vi "Initialize_etc.vi"(7 "큐 입력":refnum<queue>, 8 "error in":errorcluster caption="에러 입력(에러 없음)", 11 "입력 클러스터":T1) -> (0 "error out":errorcluster caption="에러 출력", 3 "data 1":string[][](array[string]), 4 "Load?":bool)   [LabVIEW 2020]
uses:
  Controls/Clst_Initialize Input.ctl
  Controls/Cmd_Var Data IO.ctl
  Variables/Global_Cal Info.vi
  Public/Polymorph/Table Initialize_2D.vi
  Public/Polymorph/Array Dedup_1D Str.vi
  Public/Polymorph/String content_Str.vi
  Public/Polymorph/String content_Combo.vi
  Public/Polymorph/Table Initialize_Str.vi
  Public/Polymorph/Cell Space_Table.vi
  Public/Polymorph/Rmv Empt Arr_2D Str.vi
  <vilib>/express/express arith-compare/Formula/XNode/ExpressFormulaBlockNode.xnode
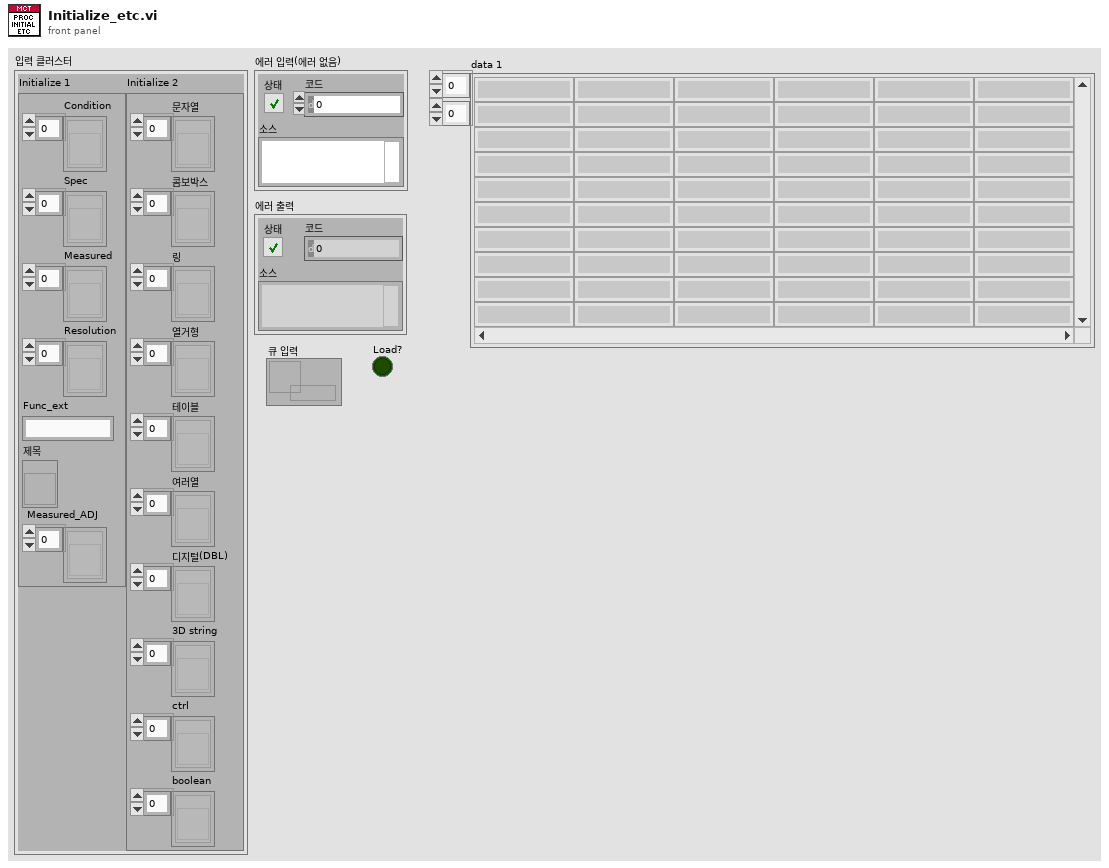
[diagram p1: front panel]
types:
  T1 = typedef "Clst_Initialize Input.ctl" = cluster{"Initialize 1":cluster{"Condition":refnum<vi>[], "Spec":refnum<vi>[], "Measured":refnum<vi>[], "Resolution":refnum<vi>[], "Func_ext":string, "제목":refnum<vi>, "Measured_ADJ":refnum<vi>[]}, "Initialize 2":cluster{"문자열":refnum<vi>[], "콤보박스":refnum<vi>[], "링":refnum<vi>[], "열거형":refnum<vi>[], "테이블":refnum<vi>[], "여러열":refnum<vi>[], "디지털(DBL)":refnum<vi>[], "3D string":refnum<vi>[], "ctrl":refnum<vi>[], "boolean":refnum<vi>[]}}
  T2 = cluster{"세부분류코드":string, "형식":string, "옵션":string, "측정기명":string, "EXCEL파일명":string, "TEMP":string}
  T3 = typedef "Cmd_Var Data IO.ctl" = enum16{"Condition", "Condition Default", "Condition_Temp", "Resolution", "Resolution Default", "Resolution Old", "Spec", "Spec Default", "Spec Old", "Spec Temp", "Result", "Result2", "Result3", "Result_Temp", "Result_ADJ", "Result_ADJ2", "STD1", "STD2", "STD3", "STD4", "STD5", "STD Temp", "CMC", "CMC Default"}
  T4 = enum8{"Enabled", "Disabled", "Disabled and Grayed Out"}
  T5 = typedef "Clst_Get Calproc.ctl" = cluster{"제목":string, "Condition":string[][], "Resolution":string[][], "Spec":string[][], "Data":string[][], "CMC":string[][], "NumRows":u32, "Temp_1":string[][]}
  T6 = typedef "Clst_Atm Info Global.ctl" = cluster{"교정장소":enum16{"0 : 고정표준실", "1 : 현장교정"}, "최저온도(℃)":string, "최고온도(℃)":string, "최저습도(％ R.H.)":string, "최고습도(％ R.H.)":string, "최저기압(hPa)":string, "최고기압(hPa)":string, "교정실명":string}
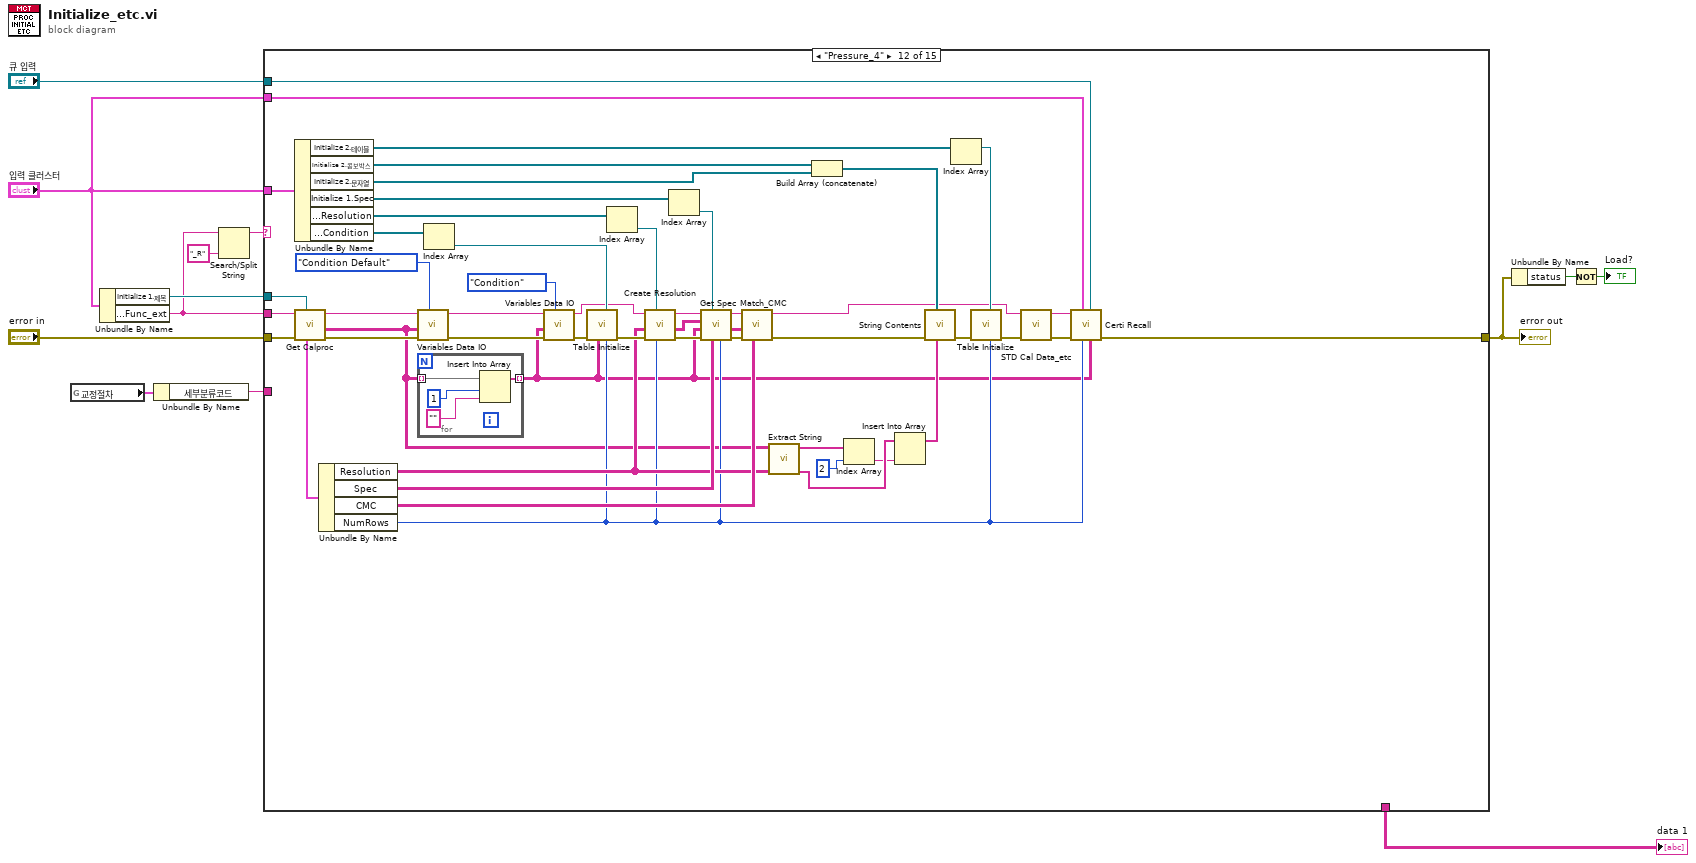
[diagram p0: block diagram]
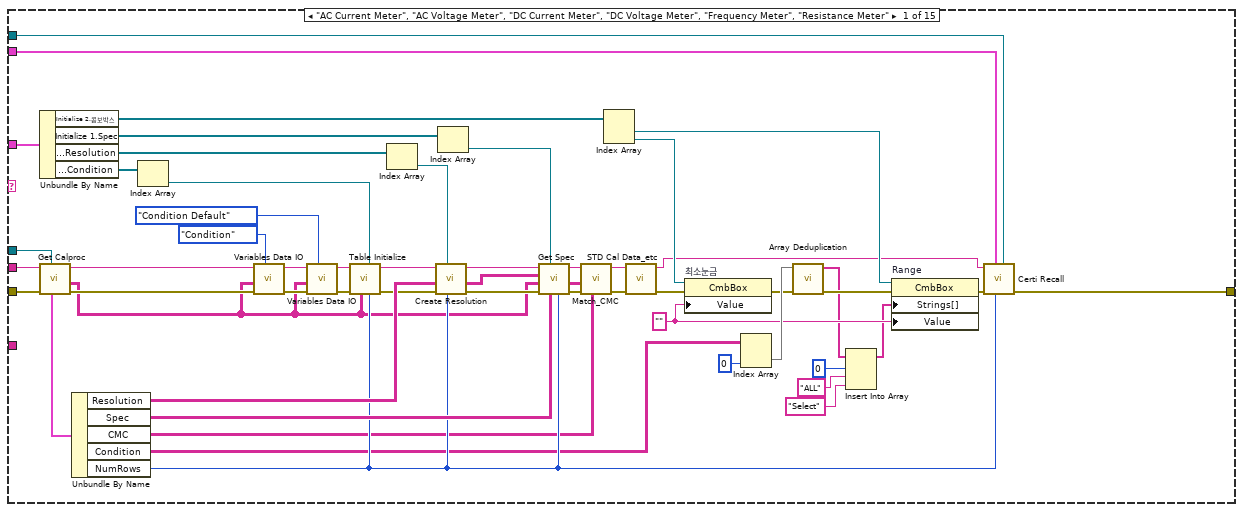
[diagram p2: hidden frame]
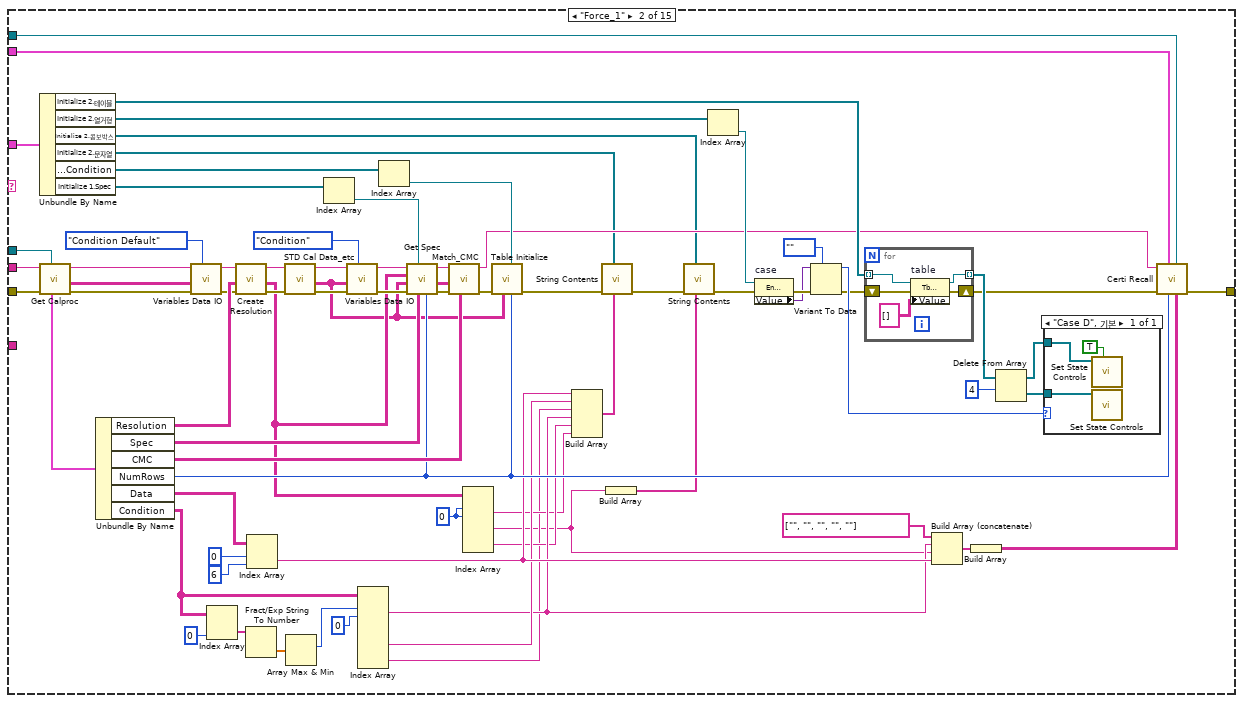
[diagram p3: hidden frame]
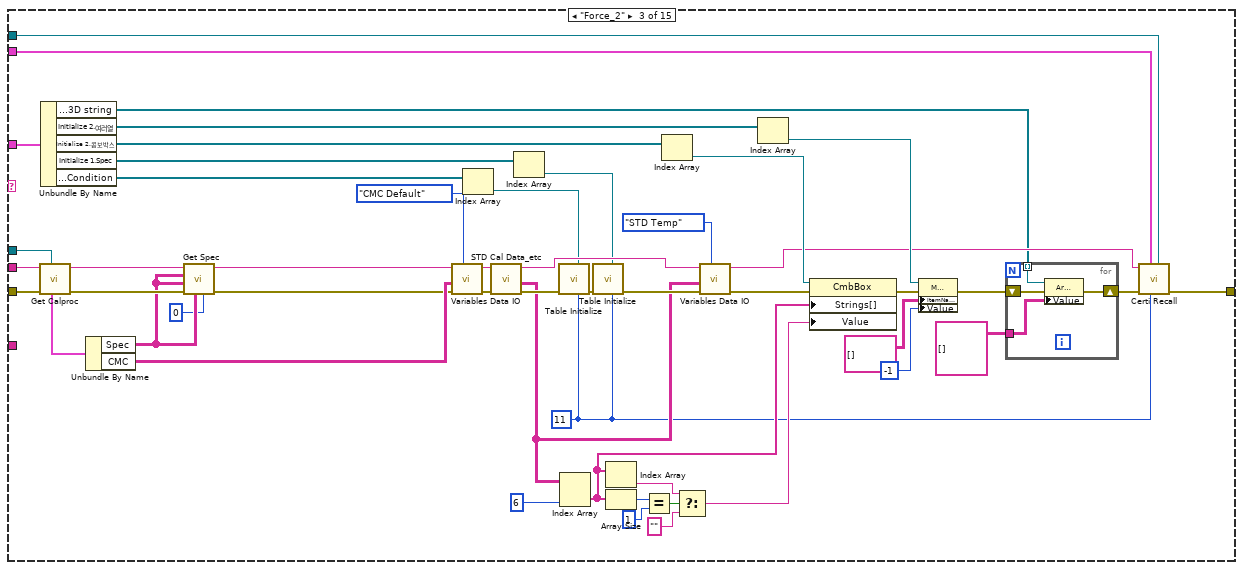
[diagram p4: hidden frame]
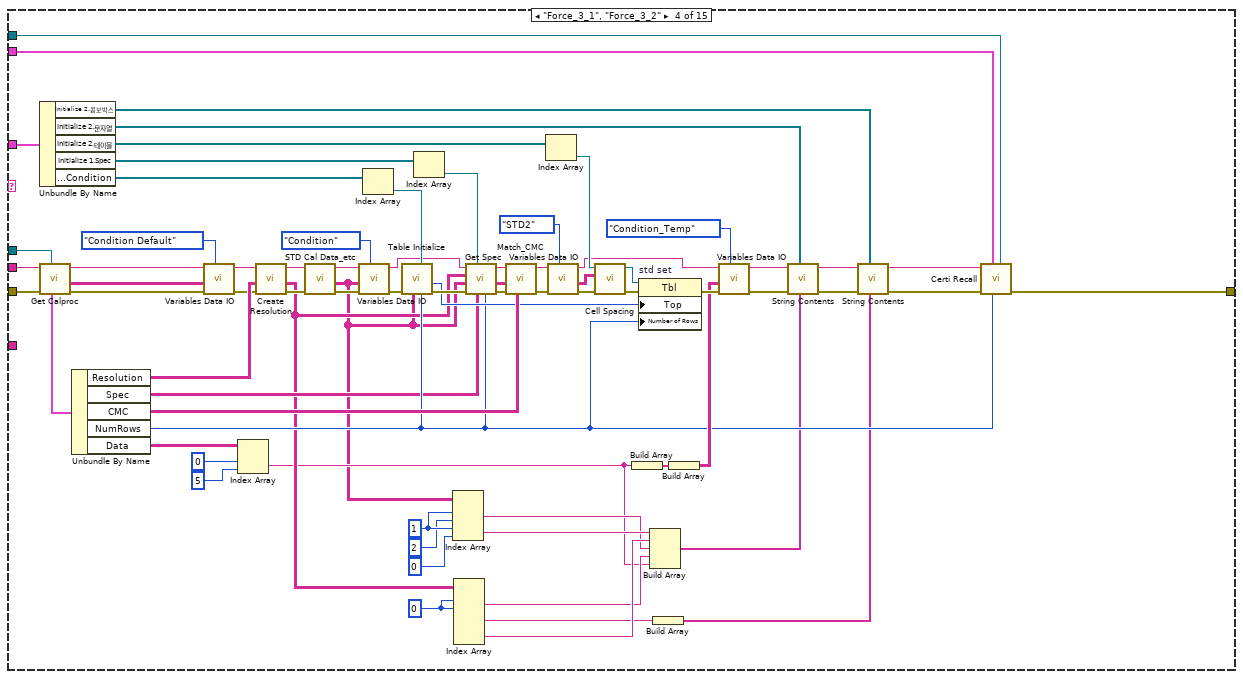
[diagram p5: hidden frame]
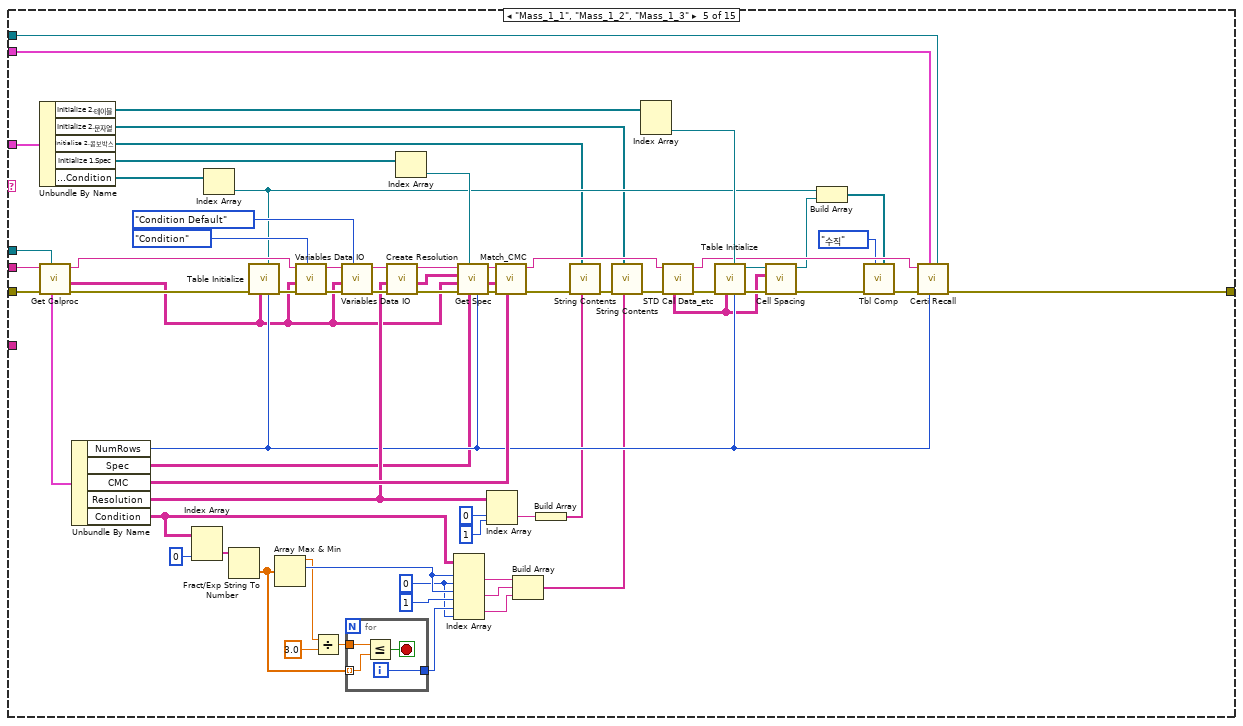
[diagram p6: hidden frame]
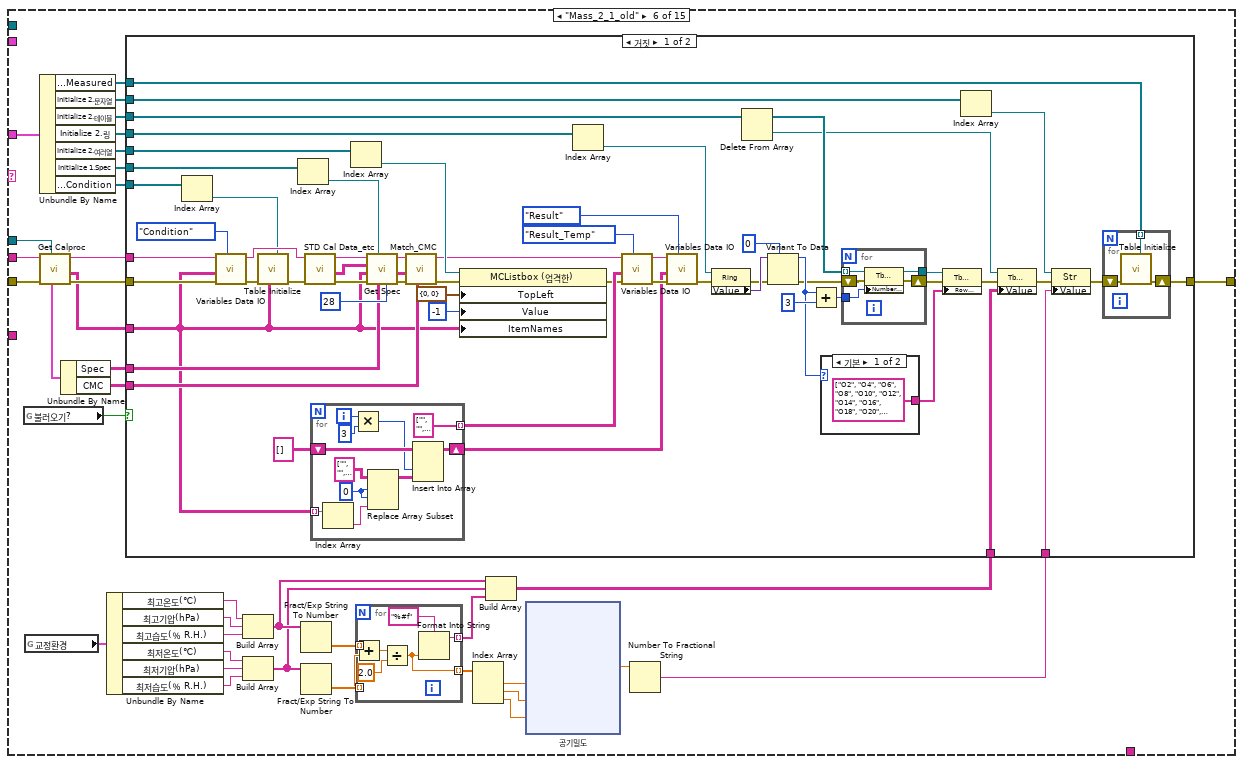
[diagram p7: hidden frame]
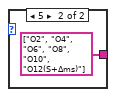
[diagram p8: hidden frame]
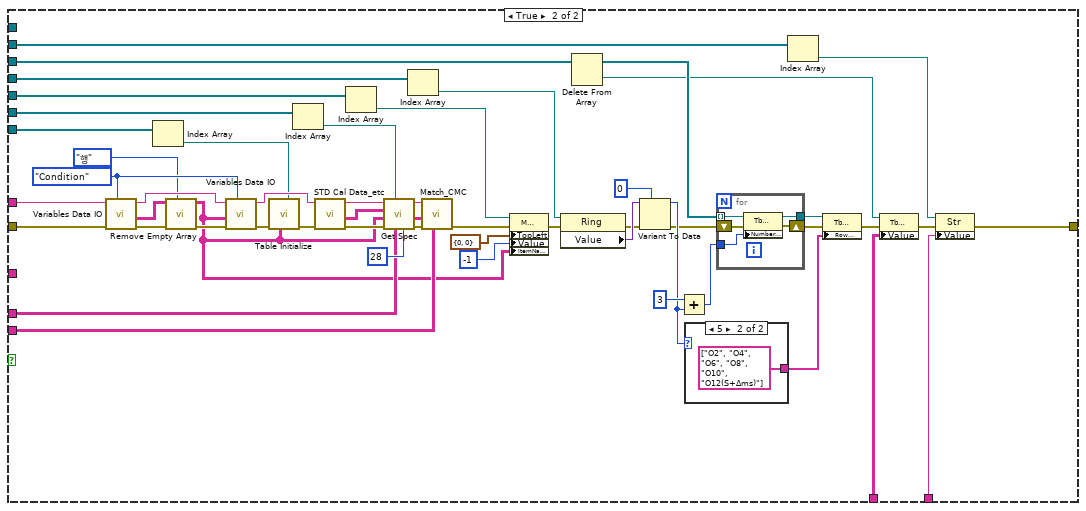
[diagram p9: hidden frame]
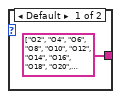
[diagram p10: hidden frame]
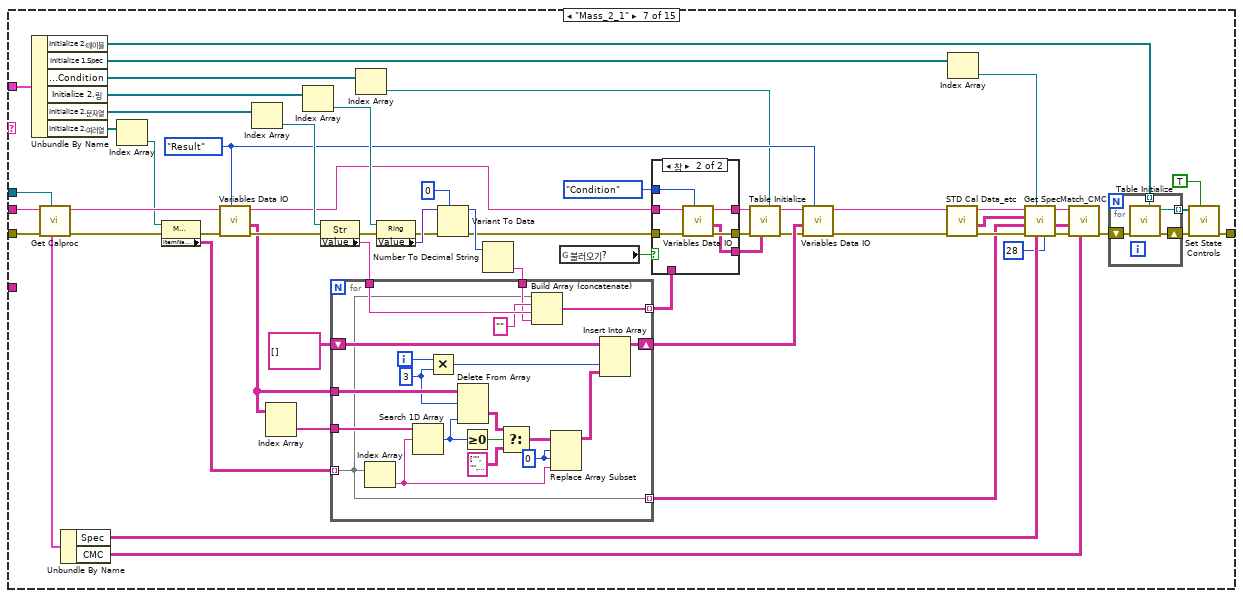
[diagram p11: hidden frame]
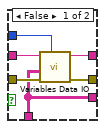
[diagram p12: hidden frame]
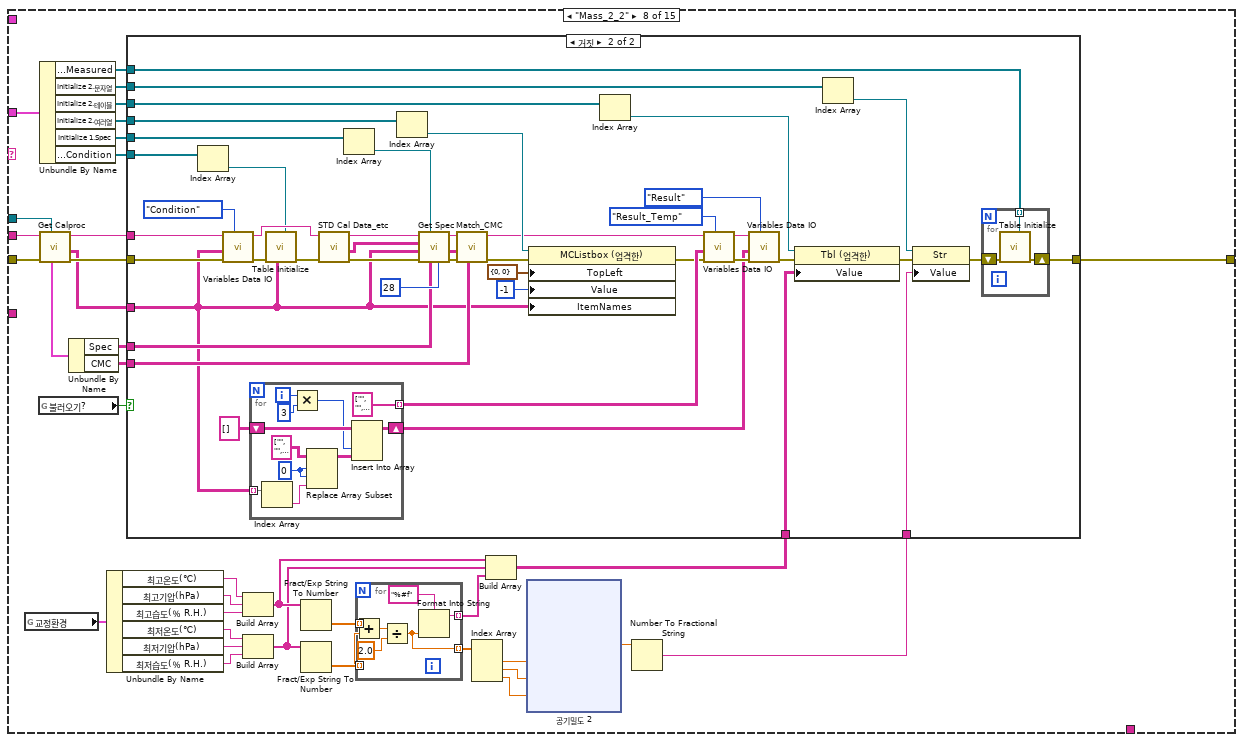
[diagram p13: hidden frame]
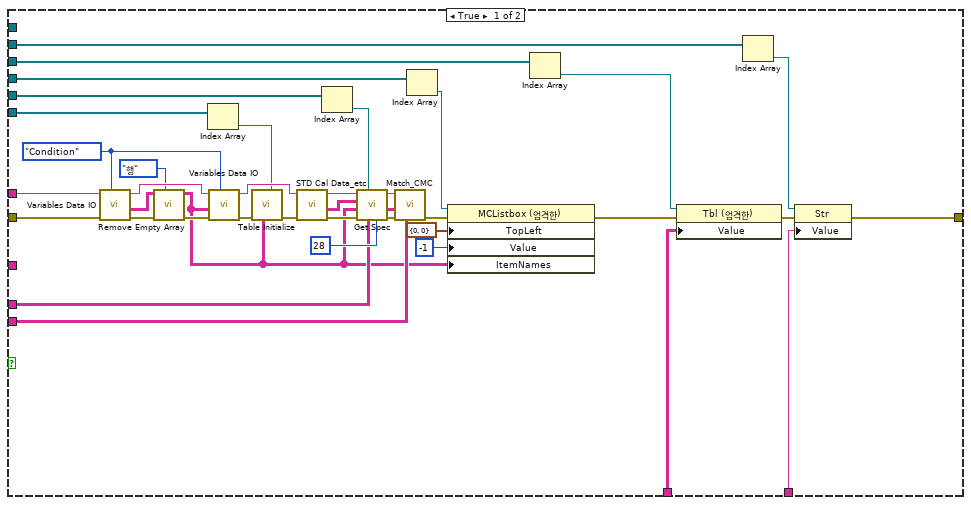
[diagram p14: hidden frame]
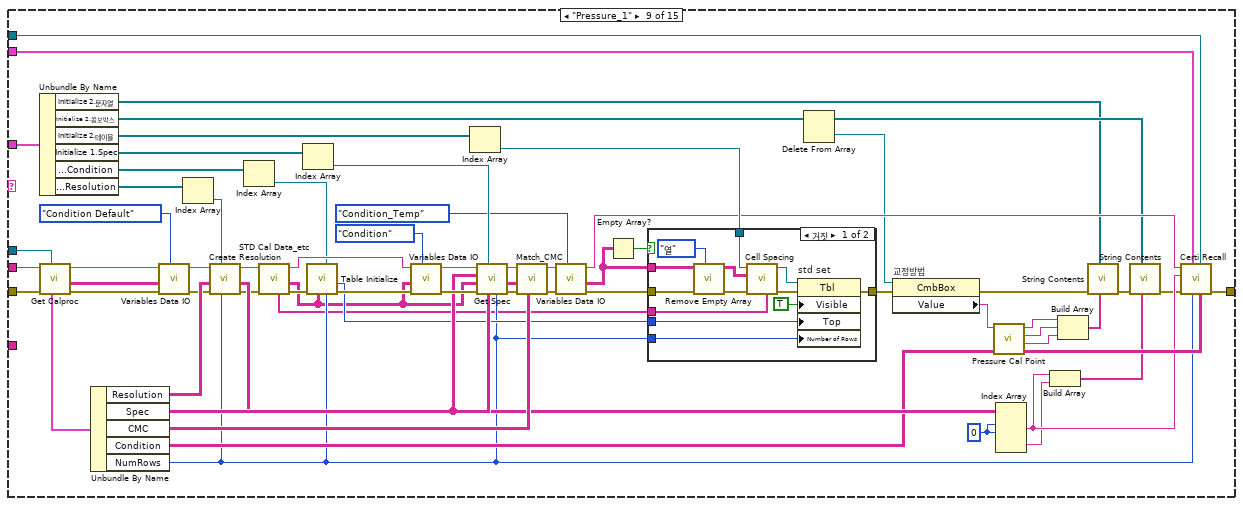
[diagram p15: hidden frame]
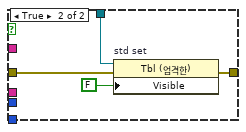
[diagram p16: hidden frame]
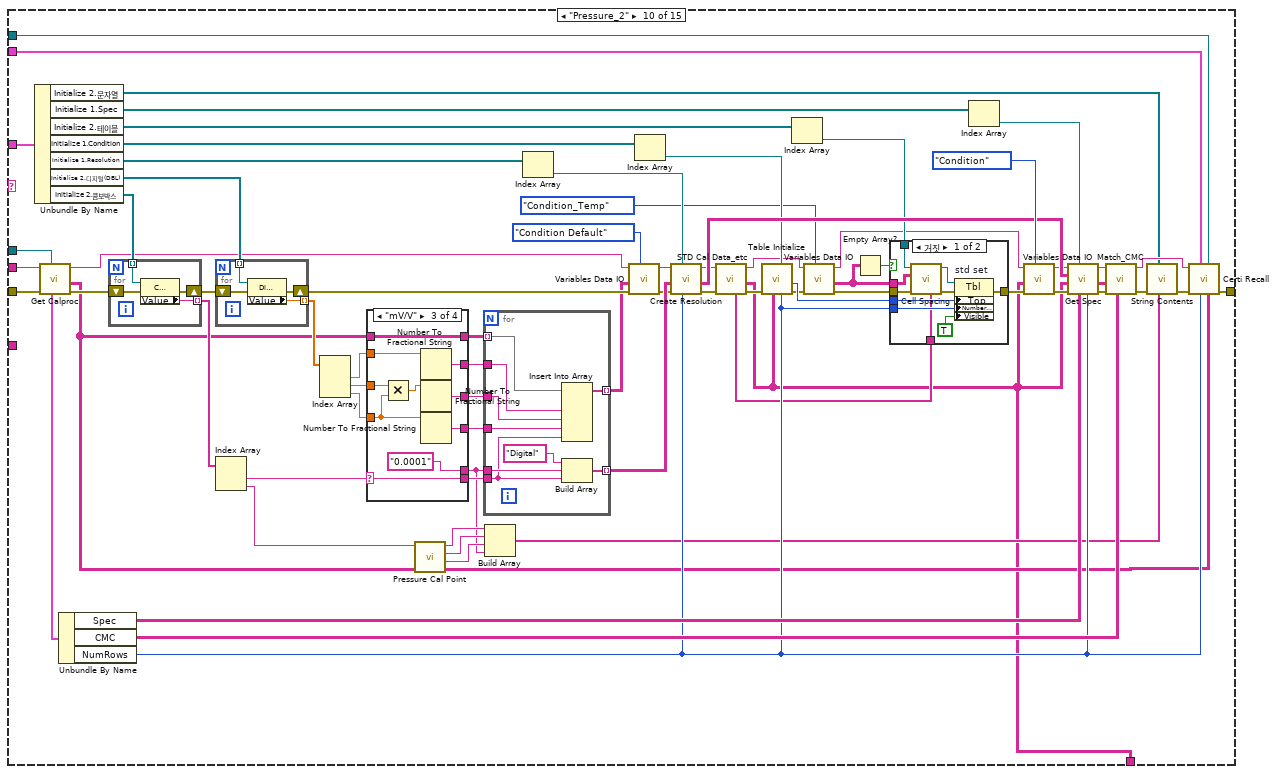
[diagram p17: hidden frame]
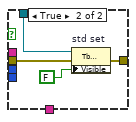
[diagram p18: hidden frame]
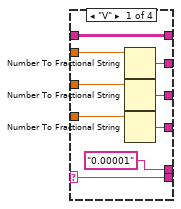
[diagram p19: hidden frame]
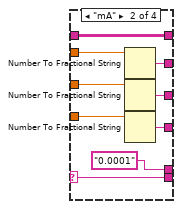
[diagram p20: hidden frame]
diagram:
  n1 = global read "Global_Cal Info.vi" "교정절차"() -> (w11:T2)
  n2 = Unbundle By Name("입력 클러스터") -> ("Initialize 1.제목"=w9:refnum<vi>, "Initialize 1.Func_ext"=w4:string)
  n3 = Unbundle By Name(w11) -> ("세부분류코드"=w10:string)
  n4 = Search/Split String(string=w4, search string/char (-)="_R" ("검색 문자열/문자 (-)")) -> (substring before match=w3:string)  [unwired: 1 in, 2 out]
  n5 = case shown="\"Pressure_4\"" w3 {
    tunnel: "error in" -> [w66 w141 w199 w274 w342 w384 w601 w674 w858 w949 w1090 w1140 w1205 w1271 w1287]
    tunnel: [w25 w74 w163 w225 w307 w360 w590 w651 w837 w917 w1063 w1128 w1174 w1257 w1287] -> w8
    tunnel: "입력 클러스터" -> [w24 w115 w170 w244 w343 w385 w602 w675 w859 w950 w1091 w1141 w1206 w1272 _]
    tunnel: [_ _ _ _ _ _ _ _ _ w877 _ _ _ w1207 string[][] [] ("CMC Out")] -> w13
    tunnel: "큐 입력" -> [w34 w104 w165 w227 w306 _ _ _ w836 w930 w1066 w1130 w1173 w1258 _]
    tunnel: w4 -> [w37 w133 w198 w263 w311 w354 w594 w645 w840 w937 w1075 w1133 w1194 w1260 _]
    tunnel: w10 -> [_ _ _ _ _ _ _ _ _ _ _ _ _ _ _]
    tunnel: "입력 클러스터" -> [w23 w103 w164 w226 w305 _ _ _ w835 w929 w1064 w1129 w1172 w1256 _]
    tunnel: w9 -> [w18 w89 w161 w218 w298 w352 w592 w643 w824 w921 w1054 w1125 w1163 w1253 _]
    frame "AC Current Meter", "AC Voltage Meter", "DC Current Meter", "DC Voltage Meter", "Frequency Meter", "Resistance Meter" {
      w51 = "" ("값")
      n6 = Unbundle By Name(w24) -> ("Initialize 2.콤보박스"=w63:refnum<vi>[], "Initialize 1.Spec"=w28:refnum<vi>[], "Initialize 1.Resolution"=w29:refnum<vi>[], "Initialize 1.Condition"=w65:refnum<vi>[])
      n7 = call "Get Calproc.vi"("제목"=w18, "에러 입력"=w66, "Func_ext"=w37) -> ("에러 출력"=w64:errorcluster, "Condition"=w14:string[][], "Func_ext Out"=w39:string, "클러스터"=w32:T5)  [unwired: 5 in]
      n8 = Unbundle By Name(w32) -> ("Resolution"=w40:string[][], "Spec"=w22:string[][], "CMC"=w16:string[][], "Condition"=w15:string[][], "NumRows"=w17:u32)
      n9 = Index Array(array=w65) -> (element=w35:refnum<vi>)  [unwired: 1 in]
      n10 = call "Variables Data IO.vi"("Select"=Cmd_Var_Data_IO."Condition", "error in"=w64, "Data In"=w14, "Func_ext"=w39) -> ("error out"=w61:errorcluster, "Func_ext Out"=w43:string)  [unwired: 5 in, 1 out]
      n11 = call "Variables Data IO.vi"("Select"=Cmd_Var_Data_IO."Condition Default", "error in"=w61, "Data In"=w14, "Func_ext"=w43) -> ("error out"=w31:errorcluster, "Func_ext Out"=w42:string)  [unwired: 5 in, 1 out]
      n12 = call-poly "Table Initialize.vi"("행의 개수"=w17, "Table Ref"=w35, "Value"=w14, "에러 입력"=w31) -> ("에러 출력"=w30:errorcluster)  [unwired: 5 in, 2 out]
      n13 = Index Array(array=w29) -> (element=w19:refnum<vi>)  [unwired: 1 in]
      n14 = call "Create Resolution.vi"("행의 개수"=w17, "Table Ref"=w19, "에러 입력(에러 없음)"=w30, "Resolution"=w40, "Func_ext"=w42) -> ("에러 출력"=w44:errorcluster, "Resolution Out"=w21:string[][], "Func_ext 출력"=w20:string)  [unwired: 4 in]
      n15 = Index Array(array=w28) -> (element=w50:refnum<vi>)  [unwired: 1 in]
      n16 = call "Get Spec.vi"("NumRows"=w17, "Spec in"=w22, "Spec Ref."=w50, "error in"=w44, "Condition in"=w14, "Resolution in"=w21, "Func_ext"=w20) -> ("error out"=w59:errorcluster, "Data Out"=w36:string[][], "Func_ext Out"=w41:string)  [unwired: 2 out]
      n17 = call "Match_CMC.vi"("CMC IN"=w16, "error in"=w59, "Condition IN"=w36, "Func_ext"=w41) -> ("error out"=w58:errorcluster, "Func_ext out"=w38:string)  [unwired: 4 in, 2 out]
      n18 = Index Array(array=w63) -> (element #1=w55:refnum<vi>, element #2=w57:refnum<vi>)  [unwired: 2 in]
      n19 = call "STD Cal Data_etc.vi"("error in"=w58, "Func_ext"=w38) -> ("error out"=w27:errorcluster, "Func_ext Out"=w33:string)  [unwired: 5 in, 3 out]
      n20 = property on="최소눈금" class="CmbBox"(reference=w57, error in=w27, "Value"=w51) -> (error out=w53:errorcluster)  [unwired: 1 out]
      n21 = Index Array(array=w15, index (col)=0 ("비활성화된 인덱스 (열)")) -> (element=w54:string[])  [unwired: 1 in]
      n22 = call-poly "Array Deduplication.vi"("error in (no error)"=w53, "배열 in"=w54) -> ("error out"=w52:errorcluster, "배열 out"=w46:string[])  [unwired: 8 in]
      n23 = Insert Into Array(array=w46, index=0 ("인덱스"), new element #1="ALL" ("새 원소/부분배열"), new element #2="Select" ("새 원소/부분배열")) -> (w45:string[])
      n24 = property on="Range" class="CmbBox"(reference=w55, error in=w52, "Strings[]"=w45, "Value"=w51) -> (error out=w26:errorcluster)  [unwired: 1 out]
      n25 = call "Certi Recall.vi"("큐 입력"=w34, "NumRows"=w17, "입력 클러스터"=w23, "에러 입력"=w26, "Func_ext in"=w33) -> ("에러 출력"=w25:errorcluster)  [unwired: 5 in, 1 out]
    }
    frame "Force_1" {
      w111 = 0 ("인덱스 (행)")
      n26 = Unbundle By Name(w115) -> ("Initialize 2.테이블"=w112:refnum<vi>[], "Initialize 2.열거형"=w100:refnum<vi>[], "Initialize 2.콤보박스"=w68:refnum<vi>[], "Initialize 2.문자열"=w76:refnum<vi>[], "Initialize 1.Condition"=w131:refnum<vi>[], "Initialize 1.Spec"=w96:refnum<vi>[])
      n27 = call "Get Calproc.vi"("제목"=w89, "에러 입력"=w141, "Func_ext"=w133) -> ("에러 출력"=w140:errorcluster, "Condition"=w88:string[][], "Func_ext Out"=w136:string, "클러스터"=w107:T5)  [unwired: 5 in]
      n28 = Unbundle By Name(w107) -> ("Resolution"=w130:string[][], "Spec"=w92:string[][], "CMC"=w135:string[][], "NumRows"=w98:u32, "Data"=w110:string[][], "Condition"=w87:string[][])
      n29 = call "Variables Data IO.vi"("Select"=Cmd_Var_Data_IO."Condition Default", "error in"=w140, "Data In"=w88, "Func_ext"=w136) -> ("error out"=w129:errorcluster, "Func_ext Out"=w126:string)  [unwired: 5 in, 1 out]
      n30 = Index Array(array=w87, index (col)=0 ("비활성화된 인덱스 (열)")) -> (element=w122:string[])  [unwired: 1 in]
      n31 = call "Create Resolution.vi"("에러 입력(에러 없음)"=w129, "Resolution"=w130, "Func_ext"=w126) -> ("에러 출력"=w128:errorcluster, "Resolution Out"=w91:string[][], "Func_ext 출력"=w125:string)  [unwired: 6 in]
      n32 = Fract/Exp String To Number(string=w122) -> (number=w121:dbl[])  [unwired: 3 in, 1 out]
      n33 = Index Array(array=w110, index (row)=0 ("인덱스 (행)"), index (col)=6 ("비활성화된 인덱스 (열)")) -> (element=w82:string)
      n34 = call "STD Cal Data_etc.vi"("error in"=w128, "Func_ext"=w125) -> ("error out"=w127:errorcluster, "Data Out"=w72:string[][], "Func_ext Out"=w124:string)  [unwired: 5 in, 2 out]
      n35 = Array Max & Min(array=w121) -> (max index (indices)=w120:i32)  [unwired: 3 out]
      n36 = Index Array(array=w96) -> (element=w138:refnum<vi>)  [unwired: 1 in]
      n37 = call "Variables Data IO.vi"("Select"=Cmd_Var_Data_IO."Condition", "error in"=w127, "Data In"=w72, "Func_ext"=w124) -> ("error out"=w97:errorcluster, "Func_ext Out"=w90:string)  [unwired: 5 in, 1 out]
      n38 = Index Array(array=w87, index (row) #1=w120, index (col) #1=0 ("비활성화된 인덱스 (열)")) -> (element #1=w80:string, element #3=w81:string, element #4=w75:string)  [unwired: 6 in, 1 out]
      n39 = Index Array(array=w131) -> (element=w123:refnum<vi>)  [unwired: 1 in]
      n40 = call "Get Spec.vi"("NumRows"=w98, "Spec in"=w92, "Spec Ref."=w138, "error in"=w97, "Condition in"=w72, "Resolution in"=w91, "Func_ext"=w90) -> ("error out"=w95:errorcluster, "Data Out"=w132:string[][], "Func_ext Out"=w137:string)  [unwired: 2 out]
      n41 = call "Match_CMC.vi"("CMC IN"=w135, "error in"=w95, "Condition IN"=w132, "Func_ext"=w137) -> ("error out"=w94:errorcluster, "Func_ext out"=w102:string)  [unwired: 4 in, 2 out]
      n42 = Index Array(array=w91, index (row) #1=w111, index (col) #1=w111) -> (element #1=w78:string, element #2=w71:string, element #3=w79:string)  [unwired: 4 in]
      n43 = call-poly "Table Initialize.vi"("행의 개수"=w98, "Table Ref"=w123, "Value"=w72, "에러 입력"=w94) -> ("에러 출력"=w93:errorcluster)  [unwired: 5 in, 2 out]
      n44 = Build Array(w82, w81, w75, w80, w79, w78) -> (w77:string[])
      n45 = call-poly "String Contents.vi"("문자 배열"=w77, "참조 배열"=w76, "에러 입력"=w93) -> ("에러 출력"=w70:errorcluster)  [unwired: 7 in, 1 out]
      n46 = Build Array(w71) -> (w67:string[])
      n47 = call-poly "String Contents.vi"("문자 배열"=w67, "참조 배열"=w68, "에러 입력"=w70) -> ("에러 출력"=w69:errorcluster)  [unwired: 7 in, 1 out]
      n48 = Index Array(array=w100) -> (element=w113:refnum<vi>)  [unwired: 1 in]
      n49 = property on="case" class="Enum"(reference=w113, error in=w69) -> (error out=w118:errorcluster, "Value"=w117:variant)  [unwired: 1 out]
      n50 = Variant To Data(error in=w118, type=enum16{"", "Case B", "Case D"}."" ("Case"), Variant=w117) -> (data=w114:enum16{"", "Case B", "Case D"}, error out=w73:errorcluster)
      n51 = for {
        tunnel: w112 -> [w146] mode=indexing
        tunnel: [w144] -> w86 mode=indexing
        shift-right: [w142] -> _
        shift-left: w73 -> [w143]
        n52 = property on="table" class="Tbl (엄격한)"(reference=w146, error in=w143, "Value"=string[][] [] ("값")) -> (reference out=w144:refnum<vi>, error out=w142:errorcluster)
      }
      n53 = Build Array (concatenate)(string[] ["", "", "", "", ""], w80, w71, w82) -> (w106:string[])
      n54 = Build Array(w106) -> (w101:string[][])
      n55 = Delete From Array(array=w86, length=4 ("길이")) -> (deleted portion=w85:refnum<vi>[], array with subset deleted=w83:refnum<vi>[])  [unwired: 1 in]
      n56 = case shown="\"Case D\", 기본" w114 {
        tunnel: w85 -> [w149]
        tunnel: w83 -> [w147]
        frame "Case D", Default {
          n57 = call "Set State Controls.vi"("활성화 (F)"=TRUE, "컨트롤 참조 배열 in"=w147) -> ()  [unwired: 8 in, 2 out]
          n58 = call "Set State Controls.vi"("컨트롤 참조 배열 in"=w149) -> ()  [unwired: 9 in, 2 out]
        }
      }
      n59 = call "Certi Recall.vi"("Value"=w101, "큐 입력"=w104, "NumRows"=w98, "입력 클러스터"=w103, "에러 입력"=w73, "Func_ext in"=w102) -> ("에러 출력"=w74:errorcluster)  [unwired: 4 in, 1 out]
    }
    frame "Force_2" {
      w156 = u32 11 ("NumRows")
      n60 = call "Get Calproc.vi"("제목"=w161, "에러 입력"=w199, "Func_ext"=w198) -> ("에러 출력"=w155:errorcluster, "Func_ext Out"=w154:string, "클러스터"=w167:T5)  [unwired: 5 in, 1 out]
      n61 = Unbundle By Name(w170) -> ("Initialize 2.3D string"=w160:refnum<vi>[], "Initialize 2.여러열"=w189:refnum<vi>[], "Initialize 2.콤보박스"=w193:refnum<vi>[], "Initialize 1.Spec"=w180:refnum<vi>[], "Initialize 1.Condition"=w181:refnum<vi>[])
      n62 = Unbundle By Name(w167) -> ("Spec"=w151:string[][], "CMC"=w196:string[][])
      n63 = call "Get Spec.vi"("NumRows"=u32 0, "Spec in"=w151, "error in"=w155, "Condition in"=w151, "Resolution in"=w151, "Func_ext"=w154) -> ("error out"=w152:errorcluster, "Func_ext Out"=w153:string)  [unwired: 1 in, 3 out]
      n64 = call "Variables Data IO.vi"("Select"=Cmd_Var_Data_IO."CMC Default", "error in"=w152, "Data In"=w196, "Func_ext"=w153) -> ("error out"=w185:errorcluster, "Func_ext Out"=w184:string)  [unwired: 5 in, 1 out]
      n65 = Index Array(array=w181) -> (element=w169:refnum<vi>)  [unwired: 1 in]
      n66 = call "STD Cal Data_etc.vi"("error in"=w185, "Func_ext"=w184) -> ("error out"=w182:errorcluster, "Data Out"=w162:string[][], "Func_ext Out"=w183:string)  [unwired: 5 in, 2 out]
      n67 = Index Array(array=w180) -> (element=w168:refnum<vi>)  [unwired: 1 in]
      n68 = call-poly "Table Initialize.vi"("행의 개수"=w156, "Table Ref"=w169, "에러 입력"=w182) -> ("에러 출력"=w195:errorcluster)  [unwired: 6 in, 2 out]
      n69 = Index Array(array=w162, index (col)=6 ("비활성화된 인덱스 (열)")) -> (element=w175:string[])  [unwired: 1 in]
      n70 = call-poly "Table Initialize.vi"("행의 개수"=w156, "Table Ref"=w168, "에러 입력"=w195) -> ("에러 출력"=w179:errorcluster)  [unwired: 6 in, 2 out]
      n71 = Index Array(array=w175) -> (element=w174:string)  [unwired: 1 in]
      n72 = Array Size(array=w175) -> (size(s)=w178:i32)
      n73 = Equal?(x=w178, y=1) -> (x = y?=w176:bool)
      n74 = Index Array(array=w193) -> (element=w191:refnum<vi>)  [unwired: 1 in]
      n75 = Select(t=w174, s=w176, f="") -> (s? t:f=w173:string)
      n76 = call "Variables Data IO.vi"("Select"=Cmd_Var_Data_IO."STD Temp", "error in"=w179, "Data In"=w162, "Func_ext"=w183) -> ("error out"=w192:errorcluster, "Func_ext Out"=w166:string)  [unwired: 5 in, 1 out]
      n77 = Index Array(array=w189) -> (element=w187:refnum<vi>)  [unwired: 1 in]
      n78 = property class="CmbBox"(reference=w191, error in=w192, "Strings[]"=w175, "Value"=w173) -> (error out=w188:errorcluster)  [unwired: 1 out]
      n79 = property class="MCListbox (엄격한)"(reference=w187, error in=w188, "ItemNames"=string[][] [], "Value"=-1 ("값")) -> (error out=w159:errorcluster)  [unwired: 1 out]
      n80 = for {
        tunnel: w160 -> [w203] mode=indexing
        shift-right: [w201] -> w158
        shift-left: w159 -> [w202]
        tunnel: string[][][] [] -> [w200]
        n81 = property class="Arr (엄격한)"(reference=w203, error in=w202, "Value"=w200) -> (error out=w201:errorcluster)  [unwired: 1 out]
      }
      n82 = call "Certi Recall.vi"("큐 입력"=w165, "NumRows"=w156, "입력 클러스터"=w164, "에러 입력"=w158, "Func_ext in"=w166) -> ("에러 출력"=w163:errorcluster)  [unwired: 5 in, 1 out]
    }
    frame "Force_3_1", "Force_3_2" {
      w224 = 1 ("인덱스 (행)")
      w243 = 0 ("인덱스 (행)")
      n83 = Unbundle By Name(w244) -> ("Initialize 2.콤보박스"=w205:refnum<vi>[], "Initialize 2.문자열"=w216:refnum<vi>[], "Initialize 2.테이블"=w245:refnum<vi>[], "Initialize 1.Spec"=w260:refnum<vi>[], "Initialize 1.Condition"=w261:refnum<vi>[])
      n84 = call "Get Calproc.vi"("제목"=w218, "에러 입력"=w274, "Func_ext"=w263) -> ("에러 출력"=w273:errorcluster, "Condition"=w217:string[][], "Func_ext Out"=w269:string, "클러스터"=w229:T5)  [unwired: 5 in]
      n85 = Unbundle By Name(w229) -> ("Resolution"=w259:string[][], "Spec"=w221:string[][], "CMC"=w268:string[][], "NumRows"=w222:u32, "Data"=w242:string[][])
      n86 = call "Variables Data IO.vi"("Select"=Cmd_Var_Data_IO."Condition Default", "error in"=w273, "Data In"=w217, "Func_ext"=w269) -> ("error out"=w258:errorcluster, "Func_ext Out"=w255:string)  [unwired: 5 in, 1 out]
      n87 = Index Array(array=w242, index (row)=0 ("인덱스 (행)"), index (col)=5 ("비활성화된 인덱스 (열)")) -> (element=w210:string)
      n88 = call "Create Resolution.vi"("에러 입력(에러 없음)"=w258, "Resolution"=w259, "Func_ext"=w255) -> ("에러 출력"=w257:errorcluster, "Resolution Out"=w220:string[][], "Func_ext 출력"=w254:string)  [unwired: 6 in]
      n89 = call "STD Cal Data_etc.vi"("error in"=w257, "Func_ext"=w254) -> ("error out"=w256:errorcluster, "Data Out"=w209:string[][], "Func_ext Out"=w253:string)  [unwired: 5 in, 2 out]
      n90 = call "Variables Data IO.vi"("Select"=Cmd_Var_Data_IO."Condition", "error in"=w256, "Data In"=w209, "Func_ext"=w253) -> ("error out"=w265:errorcluster, "Func_ext Out"=w219:string)  [unwired: 5 in, 1 out]
      n91 = Index Array(array=w261) -> (element=w238:refnum<vi>)  [unwired: 1 in]
      n92 = call-poly "Table Initialize.vi"("행의 개수"=w222, "Table Ref"=w238, "Value"=w209, "에러 입력"=w265) -> ("에러 출력"=w239:errorcluster, "Bottom"=w237:i32)  [unwired: 5 in, 1 out]
      n93 = Index Array(array=w260) -> (element=w271:refnum<vi>)  [unwired: 1 in]
      n94 = Index Array(array=w209, index (row) #1=w224, index (col) #1=2 ("비활성화된 인덱스 (열)"), index (row) #2=w224, index (col) #2=0 ("비활성화된 인덱스 (열)")) -> (element #1=w212:string, element #2=w214:string)
      n95 = Index Array(array=w220, index (row) #1=w243, index (col) #1=w243) -> (element #1=w211:string, element #2=w208:string, element #3=w213:string)  [unwired: 4 in]
      n96 = call "Get Spec.vi"("NumRows"=w222, "Spec in"=w221, "Spec Ref."=w271, "error in"=w239, "Condition in"=w209, "Resolution in"=w220, "Func_ext"=w219) -> ("error out"=w266:errorcluster, "Data Out"=w262:string[][], "Func_ext Out"=w270:string)  [unwired: 2 out]
      n97 = call "Match_CMC.vi"("CMC IN"=w268, "error in"=w266, "Condition IN"=w262, "Func_ext"=w270) -> ("error out"=w247:errorcluster, "Func_ext out"=w251:string)  [unwired: 4 in, 2 out]
      n98 = Index Array(array=w245) -> (element=w249:refnum<vi>)  [unwired: 1 in]
      n99 = call "Variables Data IO.vi"("Select"=Cmd_Var_Data_IO."STD2", "error in"=w247, "Func_ext"=w251) -> ("error out"=w246:errorcluster, "Data Out"=w250:string[][], "Func_ext Out"=w233:string)  [unwired: 6 in]
      n100 = call-poly "Cell Spacing.vi"("error in"=w246, "Data in"=w250, "테이블 참조 in"=w249) -> ("error out"=w236:errorcluster, "테이블 참조 Out"=w248:refnum<vi>)  [unwired: 6 in, 1 out]
      n101 = Build Array(w210) -> (w231:string[])
      n102 = property on="std set" class="Tbl"(reference=w248, error in=w236, "Top"=w237, "Number of Rows"=w222) -> (error out=w235:errorcluster)  [unwired: 1 out]
      n103 = Build Array(w214, w213, w212, w211, w210) -> (w215:string[])
      n104 = Build Array(w208) -> (w204:string[])
      n105 = Build Array(w231) -> (w230:string[][])
      n106 = call "Variables Data IO.vi"("Select"=Cmd_Var_Data_IO."Condition_Temp", "error in"=w235, "Data In"=w230, "Func_ext"=w233) -> ("error out"=w234:errorcluster, "Func_ext Out"=w228:string)  [unwired: 5 in, 1 out]
      n107 = call-poly "String Contents.vi"("문자 배열"=w215, "참조 배열"=w216, "에러 입력"=w234) -> ("에러 출력"=w207:errorcluster)  [unwired: 7 in, 1 out]
      n108 = call-poly "String Contents.vi"("문자 배열"=w204, "참조 배열"=w205, "에러 입력"=w207) -> ("에러 출력"=w206:errorcluster)  [unwired: 7 in, 1 out]
      n109 = call "Certi Recall.vi"("큐 입력"=w227, "NumRows"=w222, "입력 클러스터"=w226, "에러 입력"=w206, "Func_ext in"=w228) -> ("에러 출력"=w225:errorcluster)  [unwired: 5 in, 1 out]
    }
    frame "Mass_1_1", "Mass_1_2", "Mass_1_3" {
      w328 = 0 ("비활성화된 인덱스 (열)")
      n110 = Unbundle By Name(w343) -> ("Initialize 2.테이블"=w313:refnum<vi>[], "Initialize 2.문자열"=w289:refnum<vi>[], "Initialize 2.콤보박스"=w279:refnum<vi>[], "Initialize 1.Spec"=w316:refnum<vi>[], "Initialize 1.Condition"=w341:refnum<vi>[])
      n111 = call "Get Calproc.vi"("제목"=w298, "에러 입력"=w342, "Func_ext"=w311) -> ("에러 출력"=w340:errorcluster, "Condition"=w283:string[][], "Func_ext Out"=w317:string, "클러스터"=w308:T5)  [unwired: 5 in]
      n112 = Unbundle By Name(w308) -> ("NumRows"=w303:u32, "Spec"=w302:string[][], "CMC"=w315:string[][], "Resolution"=w314:string[][], "Condition"=w297:string[][])
      n113 = Index Array(array=w297, index (col)=0 ("비활성화된 인덱스 (열)")) -> (element=w338:string[])  [unwired: 1 in]
      n114 = Index Array(array=w341) -> (element=w290:refnum<vi>)  [unwired: 1 in]
      n115 = Fract/Exp String To Number(string=w338) -> (number=w333:dbl[])  [unwired: 3 in, 1 out]
      n116 = call-poly "Table Initialize.vi"("행의 개수"=w303, "Table Ref"=w290, "Value"=w283, "에러 입력"=w340) -> ("에러 출력"=w318:errorcluster)  [unwired: 5 in, 2 out]
      n117 = Array Max & Min(array=w333) -> (max value=w332:dbl, max index (indices)=w337:i32)  [unwired: 2 out]
      n118 = call "Variables Data IO.vi"("Select"=Cmd_Var_Data_IO."Condition", "error in"=w318, "Data In"=w283, "Func_ext"=w317) -> ("error out"=w326:errorcluster, "Func_ext Out"=w321:string)  [unwired: 5 in, 1 out]
      n119 = Divide(x=w332, y=3.0) -> (x/y=w330:dbl)
      n120 = call "Variables Data IO.vi"("Select"=Cmd_Var_Data_IO."Condition Default", "error in"=w326, "Data In"=w283, "Func_ext"=w321) -> ("error out"=w323:errorcluster, "Func_ext Out"=w320:string)  [unwired: 5 in, 1 out]
      n121 = for {
        tunnel: w333 -> [w346] mode=indexing
        tunnel: w330 -> [w347]
        tunnel: [w344] -> w329
        i -> [w344]
        stop <- w345 stop-if-true
        n122 = Less Or Equal?(x=w347, y=w346) -> (x <= y?=w345:bool)
      }
      n123 = call "Create Resolution.vi"("에러 입력(에러 없음)"=w323, "Resolution"=w314, "Func_ext"=w320) -> ("에러 출력"=w322:errorcluster, "Resolution Out"=w301:string[][], "Func_ext 출력"=w300:string)  [unwired: 6 in]
      n124 = Index Array(array=w316) -> (element=w292:refnum<vi>)  [unwired: 1 in]
      n125 = Index Array(array=w297, index (row) #1=w337, index (col) #1=w328, index (row) #2=w337, index (col) #2=1 ("비활성화된 인덱스 (열)"), index (row) #3=w329, index (col) #3=w328) -> (element #1=w288:string, element #2=w287:string, element #3=w286:string)
      n126 = call "Get Spec.vi"("NumRows"=w303, "Spec in"=w302, "Spec Ref."=w292, "error in"=w322, "Condition in"=w283, "Resolution in"=w301, "Func_ext"=w300) -> ("error out"=w324:errorcluster, "Data Out"=w310:string[][], "Func_ext Out"=w319:string)  [unwired: 2 out]
      n127 = Index Array(array=w314, index (row)=0 ("인덱스 (행)"), index (col)=1 ("비활성화된 인덱스 (열)")) -> (element=w278:string)
      n128 = call "Match_CMC.vi"("CMC IN"=w315, "error in"=w324, "Condition IN"=w310, "Func_ext"=w319) -> ("error out"=w280:errorcluster, "Func_ext out"=w291:string)  [unwired: 4 in, 2 out]
      n129 = Build Array(w288, w287, w286) -> (w285:string[])
      n130 = Build Array(w278) -> (w277:string[])
      n131 = call-poly "String Contents.vi"("문자 배열"=w277, "참조 배열"=w279, "에러 입력"=w280) -> ("에러 출력"=w276:errorcluster)  [unwired: 7 in, 1 out]
      n132 = call-poly "String Contents.vi"("문자 배열"=w285, "참조 배열"=w289, "에러 입력"=w276) -> ("에러 출력"=w284:errorcluster)  [unwired: 7 in, 1 out]
      n133 = Index Array(array=w313) -> (element #2=w309:refnum<vi>)  [unwired: 2 in, 1 out]
      n134 = call "STD Cal Data_etc.vi"("error in"=w284, "Func_ext"=w291) -> ("error out"=w299:errorcluster, "Func_ext Out"=w304:string, "Cal STD"=w282:string[][])  [unwired: 5 in, 2 out]
      n135 = call-poly "Table Initialize.vi"("행의 개수"=w303, "Table Ref"=w309, "Value"=w282, "에러 입력"=w299) -> ("에러 출력"=w312:errorcluster, "Table Ref out"=w275:refnum<vi>)  [unwired: 5 in, 1 out]
      n136 = call-poly "Cell Spacing.vi"("error in"=w312, "Data in"=w282, "테이블 참조 in"=w275) -> ("error out"=w296:errorcluster, "테이블 참조 Out"=w293:refnum<vi>)  [unwired: 6 in, 1 out]
      n137 = Build Array(w290, w293) -> (w281:refnum<vi>[])
      n138 = call "Tbl Comp.vi"("배열"=w281, "방향"=enum16{"수직", "수평"}."수직", "에러 입력"=w296) -> ("에러 출력"=w295:errorcluster)  [unwired: 6 in, 2 out]
      n139 = call "Certi Recall.vi"("큐 입력"=w306, "NumRows"=w303, "입력 클러스터"=w305, "에러 입력"=w295, "Func_ext in"=w304) -> ("에러 출력"=w307:errorcluster)  [unwired: 5 in, 1 out]
    }
    frame "Mass_2_1_old" {
      n140 = global read "Global_Cal Info.vi" "불러오기?"() -> (w355:bool)
      n141 = global read "Global_Cal Info.vi" "교정환경"() -> (w380:T6)
      n142 = Unbundle By Name(w385) -> ("Initialize 1.Measured"=w379:refnum<vi>[], "Initialize 2.문자열"=w348:refnum<vi>[], "Initialize 2.테이블"=w381:refnum<vi>[], "Initialize 2.링"=w361:refnum<vi>[], "Initialize 2.여러열"=w383:refnum<vi>[], "Initialize 1.Spec"=w378:refnum<vi>[], "Initialize 1.Condition"=w382:refnum<vi>[])
      n143 = call "Get Calproc.vi"("제목"=w352, "에러 입력"=w384, "Func_ext"=w354) -> ("에러 출력"=w359:errorcluster, "Condition"=w351:string[][], "Func_ext Out"=w358:string, "클러스터"=w353:T5)  [unwired: 5 in]
      n144 = Unbundle By Name(w353) -> ("Spec"=w357:string[][], "CMC"=w356:string[][])
      n145 = Unbundle By Name(w380) -> ("최고온도(℃)"=w369:string, "최고기압(hPa)"=w368:string, "최고습도(％ R.H.)"=w366:string, "최저온도(℃)"=w367:string, "최저기압(hPa)"=w377:string, "최저습도(％ R.H.)"=w376:string)
      n146 = Build Array(w369, w368, w366) -> (w365:string[])
      n147 = Build Array(w367, w377, w376) -> (w364:string[])
      n148 = Fract/Exp String To Number(string=w365) -> (number=w375:dbl[])  [unwired: 3 in, 1 out]
      n149 = Fract/Exp String To Number(string=w364) -> (number=w374:dbl[])  [unwired: 3 in, 1 out]
      n150 = for {
        tunnel: w375 -> [w531] mode=indexing
        tunnel: w374 -> [w530] mode=indexing
        tunnel: [w526] -> w363 mode=indexing
        tunnel: [w525] -> w373 mode=indexing
        n151 = Add(x=w531, y=w530) -> (x+y=w529:dbl)
        n152 = Divide(x=w529, y=2.0) -> (x/y=w525:dbl)
        n153 = Format Into String(format string="%#f" ("포맷 문자열"), w525) -> (resulting string=w526:string)  [unwired: 2 in, 1 out]
      }
      n154 = Index Array(array=w373) -> (element #1=w372:dbl, element #2=w371:dbl, element #3=w370:dbl)  [unwired: 3 in]
      n155 = Build Array(w365, w364, w363) -> (w362:string[][])
      n156 = xnode ("공기밀도")("t"=w372, "p"=w371, "h"=w370) -> ("결과"=w349:dbl)  [unwired: 1 in, 1 out]
      n157 = Number To Fractional String(number=w349) -> (F-format string=w350:string)  [unwired: 3 in]
      n158 = case shown="거짓" w355 {
        tunnel: w383 -> [w443 w517]
        tunnel: w382 -> [w442 w516]
        tunnel: w381 -> [w393 w474]
        tunnel: w379 -> [w441 _]
        tunnel: w378 -> [w440 w515]
        tunnel: w348 -> [w439 w514]
        tunnel: w362 -> [w438 w513]
        tunnel: w361 -> [w437 w512]
        tunnel: [w436 w466] -> w360
        tunnel: w359 -> [w426 w477]
        tunnel: w358 -> [w433 w486]
        tunnel: w357 -> [w400 w480]
        tunnel: w356 -> [w427 w505]
        tunnel: w351 -> [w386 _]
        tunnel: w350 -> [w397 w476]
        frame False {
          n159 = Index Array(array=w442) -> (element=w402:refnum<vi>)  [unwired: 1 in]
          n160 = call "Variables Data IO.vi"("Select"=Cmd_Var_Data_IO."Condition", "error in"=w426, "Data In"=w386, "Func_ext"=w433) -> ("error out"=w425:errorcluster, "Func_ext Out"=w432:string)  [unwired: 5 in, 1 out]
          n161 = call-poly "Table Initialize.vi"("Table Ref"=w402, "Value"=w386, "에러 입력"=w425) -> ("에러 출력"=w424:errorcluster)  [unwired: 6 in, 2 out]
          n162 = Index Array(array=w440) -> (element=w430:refnum<vi>)  [unwired: 1 in]
          n163 = call "STD Cal Data_etc.vi"("error in"=w424, "Func_ext"=w432) -> ("error out"=w413:errorcluster, "Data Out"=w399:string[][], "Func_ext Out"=w398:string)  [unwired: 5 in, 2 out]
          n164 = for {
            tunnel: w386 -> [w454] mode=indexing
            shift-right: [w449] -> w404
            shift-left: string[][] [] -> [w450]
            tunnel: [string[] ["", "", "", ""]] -> w405 mode=indexing
            i -> [w448]
            w452 = 0 ("인덱스 (행)")
            n165 = Index Array(array=w454) -> (element=w453:string)  [unwired: 1 in]
            n166 = Multiply(x=w448, y=3) -> (x*y=w446:i32)
            n167 = Replace Array Subset(array=string[][] [["", "", ""], ["", "", ""], ["", "", ""], ["", "", ""], ["", "", ""], ["", "", ""], ["", "", ""], ["", "", ""], ["", "", ""], ["", "", ""], ["", "", ""], ["", "", ""], ["", "", ""]], new element=w453, index (row)=w452, index (col)=w452) -> (w451:string[][])
            n168 = Insert Into Array(array=w450, index (col)=w446, new element=w451) -> (w449:string[][])  [unwired: 1 in]
          }
          n169 = Index Array(array=w443) -> (element=w435:refnum<vi>)  [unwired: 1 in]
          n170 = call "Get Spec.vi"("NumRows"=u32 28, "Spec in"=w400, "Spec Ref."=w430, "error in"=w413, "Condition in"=w386, "Resolution in"=w399, "Func_ext"=w398) -> ("error out"=w429:errorcluster, "Data Out"=w403:string[][], "Func_ext Out"=w428:string)  [unwired: 2 out]
          n171 = call "Match_CMC.vi"("CMC IN"=w427, "error in"=w429, "Condition IN"=w403, "Func_ext"=w428) -> ("error out"=w417:errorcluster, "Func_ext out"=w412:string)  [unwired: 4 in, 2 out]
          n172 = property class="MCListbox (엄격한)"(reference=w435, error in=w417, "TopLeft"=cluster{"Row":u32, "Column":u32} {"Row"=0, "Column"=0} ("왼쪽 위에 보이는 셀"), "Value"=-1 ("값"), "ItemNames"=w386) -> (error out=w395:errorcluster)  [unwired: 1 out]
          n173 = Index Array(array=w437) -> (element=w415:refnum<vi>)  [unwired: 1 in]
          n174 = call "Variables Data IO.vi"("Select"=Cmd_Var_Data_IO."Result_Temp", "error in"=w395, "Data In"=w405, "Func_ext"=w412) -> ("error out"=w409:errorcluster, "Func_ext Out"=w408:string)  [unwired: 5 in, 1 out]
          n175 = call "Variables Data IO.vi"("Select"=Cmd_Var_Data_IO."Result", "error in"=w409, "Data In"=w404, "Func_ext"=w408) -> ("error out"=w394:errorcluster)  [unwired: 5 in, 2 out]
          n176 = property class="Ring"(reference=w415, error in=w394) -> (error out=w416:errorcluster, "Value"=w422:variant)  [unwired: 1 out]
          n177 = Delete From Array(array=w393) -> (deleted portion=w391:refnum<vi>, array with subset deleted=w392:refnum<vi>[])  [unwired: 2 in]
          n178 = Variant To Data(error in=w416, type=u32 0, Variant=w422) -> (data=w419:u32, error out=w389:errorcluster)
          n179 = Add(x=w419, y=u32 3) -> (x+y=w418:u32)
          n180 = case shown="기본" w419 {
            tunnel: [string[] ["O2", "O4", "O6", "O8", "O10", "O12", "O14", "O16", "O18", "O20", "O22(S+Δms)"] ("행 헤더 문자열[]") string[] ["O2", "O4", "O6", "O8", "O10", "O12(S+Δms)"] ("행 헤더 문자열[]")] -> w411
            frame Default {
            }
            frame 5 {
            }
          }
          n181 = for {
            tunnel: w392 -> [w464] mode=indexing
            tunnel: w418 -> [w463]
            shift-right: [w461] -> w388
            shift-left: w389 -> [w462]
            tunnel: [w460] -> w390
            n182 = property class="Tbl (엄격한)"(reference=w464, error in=w462, "Number of Rows"=w463) -> (reference out=w460:refnum<vi>, error out=w461:errorcluster)
          }
          n183 = property class="Tbl (엄격한)"(reference=w390, error in=w388, "Row Headers[]"=w411) -> (error out=w387:errorcluster)  [unwired: 1 out]
          n184 = Index Array(array=w439) -> (element=w414:refnum<vi>)  [unwired: 1 in]
          n185 = property class="Tbl (엄격한)"(reference=w391, error in=w387, "Value"=w438) -> (error out=w396:errorcluster)  [unwired: 1 out]
          n186 = property class="Str"(reference=w414, "Value"=w397) -> ()  [unwired: 1 in, 2 out]
          n187 = for {
            tunnel: w441 -> [w455] mode=indexing
            shift-right: [w456] -> w436
            shift-left: w396 -> [w457]
            n188 = call-poly "Table Initialize.vi"("Table Ref"=w455, "에러 입력"=w457) -> ("에러 출력"=w456:errorcluster)  [unwired: 7 in, 2 out]
          }
        }
        frame True {
          w490 = Cmd_Var_Data_IO."Condition" ("Select")
          n189 = call "Variables Data IO.vi"("Select"=w490, "error in"=w477, "Func_ext"=w486) -> ("error out"=w489:errorcluster, "Data Out"=w487:string[][], "Func_ext Out"=w485:string)  [unwired: 6 in]
          n190 = Index Array(array=w516) -> (element=w482:refnum<vi>)  [unwired: 1 in]
          n191 = call-poly "Remove Empty Array.vi"("조건"=enum16{"행", "열", "행,열"}."행", "error in (no error)"=w489, "Data in"=w487) -> ("error out"=w488:errorcluster, "Data out"=w465:string[][])  [unwired: 7 in]
          n192 = call "Variables Data IO.vi"("Select"=w490, "error in"=w488, "Data In"=w465, "Func_ext"=w485) -> ("error out"=w504:errorcluster, "Func_ext Out"=w509:string)  [unwired: 5 in, 1 out]
          n193 = call-poly "Table Initialize.vi"("Table Ref"=w482, "Value"=w465, "에러 입력"=w504) -> ("에러 출력"=w503:errorcluster)  [unwired: 6 in, 2 out]
          n194 = Index Array(array=w515) -> (element=w508:refnum<vi>)  [unwired: 1 in]
          n195 = call "STD Cal Data_etc.vi"("error in"=w503, "Func_ext"=w509) -> ("error out"=w492:errorcluster, "Data Out"=w479:string[][], "Func_ext Out"=w478:string)  [unwired: 5 in, 2 out]
          n196 = Index Array(array=w517) -> (element=w511:refnum<vi>)  [unwired: 1 in]
          n197 = call "Get Spec.vi"("NumRows"=u32 28, "Spec in"=w480, "Spec Ref."=w508, "error in"=w492, "Condition in"=w465, "Resolution in"=w479, "Func_ext"=w478) -> ("error out"=w507:errorcluster, "Data Out"=w483:string[][], "Func_ext Out"=w506:string)  [unwired: 2 out]
          n198 = Index Array(array=w512) -> (element=w494:refnum<vi>)  [unwired: 1 in]
          n199 = call "Match_CMC.vi"("CMC IN"=w505, "error in"=w507, "Condition IN"=w483, "Func_ext"=w506) -> ("error out"=w496:errorcluster)  [unwired: 4 in, 3 out]
          n200 = property class="MCListbox (엄격한)"(reference=w511, error in=w496, "TopLeft"=cluster{"Row":u32, "Column":u32} {"Row"=0, "Column"=0} ("왼쪽 위에 보이는 셀"), "Value"=-1 ("값"), "ItemNames"=w465) -> (error out=w475:errorcluster)  [unwired: 1 out]
          n201 = property class="Ring"(reference=w494, error in=w475) -> (error out=w495:errorcluster, "Value"=w501:variant)  [unwired: 1 out]
          n202 = Delete From Array(array=w474) -> (deleted portion=w471:refnum<vi>, array with subset deleted=w473:refnum<vi>[])  [unwired: 2 in]
          n203 = Variant To Data(error in=w495, type=u32 0, Variant=w501) -> (data=w498:u32, error out=w472:errorcluster)
          n204 = Add(x=u32 3 ("y"), y=w498) -> (x+y=w497:u32)
          n205 = case shown="5" w498 {
            tunnel: [string[] ["O2", "O4", "O6", "O8", "O10", "O12", "O14", "O16", "O18", "O20", "O22(S+Δms)"] ("행 헤더 문자열[]") string[] ["O2", "O4", "O6", "O8", "O10", "O12(S+Δms)"] ("행 헤더 문자열[]")] -> w491
            frame Default {
            }
            frame 5 {
            }
          }
          n206 = for {
            tunnel: w473 -> [w524] mode=indexing
            tunnel: w497 -> [w523]
            shift-right: [w522] -> w469
            shift-left: w472 -> [w521]
            tunnel: [w520] -> w470
            n207 = property class="Tbl (엄격한)"(reference=w524, error in=w521, "Number of Rows"=w523) -> (reference out=w520:refnum<vi>, error out=w522:errorcluster)
          }
          n208 = Index Array(array=w514) -> (element=w493:refnum<vi>)  [unwired: 1 in]
          n209 = property class="Tbl (엄격한)"(reference=w470, error in=w469, "Row Headers[]"=w491) -> (error out=w468:errorcluster)  [unwired: 1 out]
          n210 = property class="Tbl (엄격한)"(reference=w471, error in=w468, "Value"=w513) -> (error out=w467:errorcluster)  [unwired: 1 out]
          n211 = property class="Str"(reference=w493, error in=w467, "Value"=w476) -> (error out=w466:errorcluster)  [unwired: 1 out]
        }
      }
    }
    frame "Mass_2_1" {
      w559 = Cmd_Var_Data_IO."Result" ("Select")
      n212 = Unbundle By Name(w602) -> ("Initialize 2.테이블"=w586:refnum<vi>[], "Initialize 1.Spec"=w599:refnum<vi>[], "Initialize 1.Condition"=w600:refnum<vi>[], "Initialize 2.링"=w588:refnum<vi>[], "Initialize 2.문자열"=w591:refnum<vi>[], "Initialize 2.여러열"=w579:refnum<vi>[])
      n213 = call "Get Calproc.vi"("제목"=w592, "에러 입력"=w601, "Func_ext"=w594) -> ("에러 출력"=w598:errorcluster, "Func_ext Out"=w597:string, "클러스터"=w593:T5)  [unwired: 5 in, 1 out]
      n214 = Unbundle By Name(w593) -> ("Spec"=w596:string[][], "CMC"=w595:string[][])
      n215 = Index Array(array=w579) -> (element=w578:refnum<vi>)  [unwired: 1 in]
      n216 = property class="MCListbox (엄격한)"(reference=w578, error in=w598) -> (error out=w570:errorcluster, "ItemNames"=w577:string[][])  [unwired: 1 out]
      n217 = call "Variables Data IO.vi"("Select"=w559, "error in"=w570, "Func_ext"=w597) -> ("error out"=w553:errorcluster, "Data Out"=w552:string[][], "Func_ext Out"=w558:string)  [unwired: 6 in]
      n218 = Index Array(array=w591) -> (element=w568:refnum<vi>)  [unwired: 1 in]
      n219 = Index Array(array=w552) -> (element=w551:string[])  [unwired: 2 in]
      n220 = Index Array(array=w588) -> (element=w565:refnum<vi>)  [unwired: 1 in]
      n221 = property class="Str"(reference=w568, error in=w553) -> (error out=w554:errorcluster, "Value"=w567:string)  [unwired: 1 out]
      n222 = Index Array(array=w600) -> (element=w545:refnum<vi>)  [unwired: 1 in]
      n223 = property class="Ring"(reference=w565, error in=w554) -> (error out=w555:errorcluster, "Value"=w564:variant)  [unwired: 1 out]
      n224 = Variant To Data(error in=w555, type=u32 0, Variant=w564) -> (data=w562:u32, error out=w556:errorcluster)
      n225 = Number To Decimal String(number=w562) -> (decimal integer string=w561:string)  [unwired: 1 in]
      n226 = for {
        tunnel: w577 -> [w615] mode=indexing
        shift-right: [w631] -> w569
        shift-left: string[][] [] -> [w632]
        tunnel: w567 -> [w629]
        tunnel: [w628] -> w566 mode=indexing
        tunnel: w561 -> [w626]
        tunnel: w552 -> [w625]
        tunnel: w551 -> [w623]
        tunnel: [w615] -> w550 mode=indexing
        i -> [w630]
        w621 = 3 ("y")
        w634 = 0 ("인덱스 (행)")
        n227 = Index Array(array=w615) -> (element=w622:string)  [unwired: 1 in]
        n228 = Search 1D Array(1D array=w623, element=w622) -> (index of element=w620:i32)  [unwired: 1 in]
        n229 = Multiply(x=w630, y=w621) -> (x*y=w624:i32)
        n230 = Delete From Array(array=w625, length=w621, index (col)=w620) -> (deleted portion=w618:string[][])  [unwired: 1 in, 1 out]
        n231 = Greater Or Equal To 0?(x=w620) -> (x >= 0?=w619:bool)
        n232 = Select(t=w618, s=w619, f=string[][] [["", "", ""], ["", "", ""], ["", "", ""], ["", "", ""], ["", "", ""], ["", "", ""], ["", "", ""], ["", "", ""], ["", "", ""], ["", "", ""], ["", "", ""], ["", "", ""], ["", "", ""]]) -> (s? t:f=w616:string[][])
        n233 = Build Array (concatenate)(w615, "", w629, w626) -> (w628:string[])
        n234 = Replace Array Subset(array=w616, new element=w622, index (row)=w634, index (col)=w634) -> (w633:string[][])
        n235 = Insert Into Array(array=w632, index (col)=w624, new element=w633) -> (w631:string[][])  [unwired: 1 in]
      }
      n236 = global read "Global_Cal Info.vi" "불러오기?"() -> (w549:bool)
      n237 = case shown="참" w549 {
        tunnel: w566 -> [w603 _]
        tunnel: w558 -> [w608 w614]
        tunnel: [w607 w613] -> w557
        tunnel: [w606 w612] -> w547
        tunnel: w556 -> [w605 w611]
        tunnel: Cmd_Var_Data_IO."Condition" ("Select") -> [w604 w610]
        tunnel: [w603 w609] -> w544
        frame False {
          n238 = call "Variables Data IO.vi"("Select"=w604, "error in"=w605, "Data In"=w603, "Func_ext"=w608) -> ("error out"=w606:errorcluster, "Func_ext Out"=w607:string)  [unwired: 5 in, 1 out]
        }
        frame True {
          n239 = call "Variables Data IO.vi"("Select"=w610, "error in"=w611, "Func_ext"=w614) -> ("error out"=w612:errorcluster, "Data Out"=w609:string[][], "Func_ext Out"=w613:string)  [unwired: 6 in]
        }
      }
      n240 = call-poly "Table Initialize.vi"("Table Ref"=w545, "Value"=w544, "에러 입력"=w547) -> ("에러 출력"=w546:errorcluster)  [unwired: 6 in, 2 out]
      n241 = call "Variables Data IO.vi"("Select"=w559, "error in"=w546, "Data In"=w569, "Func_ext"=w557) -> ("error out"=w575:errorcluster, "Func_ext Out"=w574:string)  [unwired: 5 in, 1 out]
      n242 = call "STD Cal Data_etc.vi"("error in"=w575, "Func_ext"=w574) -> ("error out"=w573:errorcluster, "Data Out"=w572:string[][], "Func_ext Out"=w571:string)  [unwired: 5 in, 2 out]
      n243 = Index Array(array=w599) -> (element=w576:refnum<vi>)  [unwired: 1 in]
      n244 = call "Get Spec.vi"("NumRows"=u32 28, "Spec in"=w596, "Spec Ref."=w576, "error in"=w573, "Condition in"=w550, "Resolution in"=w572, "Func_ext"=w571) -> ("error out"=w583:errorcluster, "Data Out"=w582:string[][], "Func_ext Out"=w581:string)  [unwired: 2 out]
      n245 = call "Match_CMC.vi"("CMC IN"=w595, "error in"=w583, "Condition IN"=w582, "Func_ext"=w581) -> ("error out"=w584:errorcluster)  [unwired: 4 in, 3 out]
      n246 = for {
        tunnel: [w638] -> w587 mode=indexing
        tunnel: w586 -> [w637] mode=indexing
        shift-right: [w635] -> w585
        shift-left: w584 -> [w636]
        n247 = call-poly "Table Initialize.vi"("Table Ref"=w637, "에러 입력"=w636) -> ("에러 출력"=w635:errorcluster, "Table Ref out"=w638:refnum<vi>)  [unwired: 7 in, 1 out]
      }
      n248 = call "Set State Controls.vi"("활성화 (F)"=TRUE, "error in (no error)"=w585, "컨트롤 참조 배열 in"=w587) -> ("error out"=w590:errorcluster)  [unwired: 7 in, 1 out]
    }
    frame "Mass_2_2" {
      n249 = global read "Global_Cal Info.vi" "교정환경"() -> (w670:T6)
      n250 = global read "Global_Cal Info.vi" "불러오기?"() -> (w646:bool)
      n251 = Unbundle By Name(w675) -> ("Initialize 1.Measured"=w669:refnum<vi>[], "Initialize 2.문자열"=w639:refnum<vi>[], "Initialize 2.테이블"=w671:refnum<vi>[], "Initialize 2.여러열"=w673:refnum<vi>[], "Initialize 1.Spec"=w668:refnum<vi>[], "Initialize 1.Condition"=w672:refnum<vi>[])
      n252 = call "Get Calproc.vi"("제목"=w643, "에러 입력"=w674, "Func_ext"=w645) -> ("에러 출력"=w650:errorcluster, "Condition"=w642:string[][], "Func_ext Out"=w649:string, "클러스터"=w644:T5)  [unwired: 5 in]
      n253 = Unbundle By Name(w644) -> ("Spec"=w648:string[][], "CMC"=w647:string[][])
      n254 = Unbundle By Name(w670) -> ("최고온도(℃)"=w659:string, "최고기압(hPa)"=w658:string, "최고습도(％ R.H.)"=w656:string, "최저온도(℃)"=w657:string, "최저기압(hPa)"=w667:string, "최저습도(％ R.H.)"=w666:string)
      n255 = Build Array(w659, w658, w656) -> (w655:string[])
      n256 = Build Array(w657, w667, w666) -> (w654:string[])
      n257 = Fract/Exp String To Number(string=w655) -> (number=w665:dbl[])  [unwired: 3 in, 1 out]
      n258 = Fract/Exp String To Number(string=w654) -> (number=w664:dbl[])  [unwired: 3 in, 1 out]
      n259 = for {
        tunnel: w665 -> [w780] mode=indexing
        tunnel: w664 -> [w779] mode=indexing
        tunnel: [w775] -> w653 mode=indexing
        tunnel: [w774] -> w663 mode=indexing
        n260 = Add(x=w780, y=w779) -> (x+y=w778:dbl)
        n261 = Divide(x=w778, y=2.0) -> (x/y=w774:dbl)
        n262 = Format Into String(format string="%#f" ("포맷 문자열"), w774) -> (resulting string=w775:string)  [unwired: 2 in, 1 out]
      }
      n263 = Index Array(array=w663) -> (element #1=w662:dbl, element #2=w661:dbl, element #3=w660:dbl)  [unwired: 3 in]
      n264 = Build Array(w655, w654, w653) -> (w652:string[][])
      n265 = xnode ("공기밀도 2")("t"=w662, "p"=w661, "h"=w660) -> ("결과"=w641:dbl)  [unwired: 1 in, 1 out]
      n266 = Number To Fractional String(number=w641) -> (F-format string=w640:string)  [unwired: 3 in]
      n267 = case shown="거짓" w646 {
        tunnel: w673 -> [w714 w759]
        tunnel: w672 -> [w713 w758]
        tunnel: w671 -> [w712 w757]
        tunnel: w669 -> [_ w756]
        tunnel: w668 -> [w710 w755]
        tunnel: w639 -> [w709 w754]
        tunnel: w652 -> [w708 w753]
        tunnel: [w677 w752] -> w651
        tunnel: w649 -> [w692 w751]
        tunnel: w648 -> [w682 w723]
        tunnel: w647 -> [w707 w750]
        tunnel: w642 -> [_ w715]
        tunnel: w650 -> [w693 w742]
        tunnel: w640 -> [w711 w720]
        frame True {
          w691 = Cmd_Var_Data_IO."Condition" ("Select")
          n268 = call "Variables Data IO.vi"("Select"=w691, "error in"=w693, "Func_ext"=w692) -> ("error out"=w689:errorcluster, "Data Out"=w687:string[][], "Func_ext Out"=w690:string)  [unwired: 6 in]
          n269 = call-poly "Remove Empty Array.vi"("조건"=enum16{"행", "열", "행,열"}."행", "error in (no error)"=w689, "Data in"=w687) -> ("error out"=w688:errorcluster, "Data out"=w676:string[][])  [unwired: 7 in]
          n270 = Index Array(array=w713) -> (element=w684:refnum<vi>)  [unwired: 1 in]
          n271 = call "Variables Data IO.vi"("Select"=w691, "error in"=w688, "Data In"=w676, "Func_ext"=w690) -> ("error out"=w700:errorcluster, "Func_ext Out"=w704:string)  [unwired: 5 in, 1 out]
          n272 = call-poly "Table Initialize.vi"("Table Ref"=w684, "Value"=w676, "에러 입력"=w700) -> ("에러 출력"=w695:errorcluster)  [unwired: 6 in, 2 out]
          n273 = call "STD Cal Data_etc.vi"("error in"=w695, "Func_ext"=w704) -> ("error out"=w696:errorcluster, "Data Out"=w681:string[][], "Func_ext Out"=w680:string)  [unwired: 5 in, 2 out]
          n274 = Index Array(array=w710) -> (element=w703:refnum<vi>)  [unwired: 1 in]
          n275 = call "Get Spec.vi"("NumRows"=u32 28, "Spec in"=w682, "Spec Ref."=w703, "error in"=w696, "Condition in"=w676, "Resolution in"=w681, "Func_ext"=w680) -> ("error out"=w702:errorcluster, "Data Out"=w685:string[][], "Func_ext Out"=w701:string)  [unwired: 2 out]
          n276 = call "Match_CMC.vi"("CMC IN"=w707, "error in"=w702, "Condition IN"=w685, "Func_ext"=w701) -> ("error out"=w698:errorcluster)  [unwired: 4 in, 3 out]
          n277 = Index Array(array=w714) -> (element=w706:refnum<vi>)  [unwired: 1 in]
          n278 = property class="MCListbox (엄격한)"(reference=w706, error in=w698, "TopLeft"=cluster{"Row":u32, "Column":u32} {"Row"=0, "Column"=0} ("왼쪽 위에 보이는 셀"), "Value"=-1 ("값"), "ItemNames"=w676) -> (error out=w679:errorcluster)  [unwired: 1 out]
          n279 = Index Array(array=w712) -> (element=w694:refnum<vi>)  [unwired: 1 in]
          n280 = property class="Tbl (엄격한)"(reference=w694, error in=w679, "Value"=w708) -> (error out=w678:errorcluster)  [unwired: 1 out]
          n281 = Index Array(array=w709) -> (element=w697:refnum<vi>)  [unwired: 1 in]
          n282 = property class="Str"(reference=w697, error in=w678, "Value"=w711) -> (error out=w677:errorcluster)  [unwired: 1 out]
        }
        frame False {
          n283 = Index Array(array=w758) -> (element=w725:refnum<vi>)  [unwired: 1 in]
          n284 = call "Variables Data IO.vi"("Select"=Cmd_Var_Data_IO."Condition", "error in"=w742, "Data In"=w715, "Func_ext"=w751) -> ("error out"=w741:errorcluster, "Func_ext Out"=w747:string)  [unwired: 5 in, 1 out]
          n285 = for {
            tunnel: w715 -> [w770] mode=indexing
            shift-right: [w765] -> w729
            shift-left: string[][] [] -> [w766]
            tunnel: [string[] ["", "", "", "", ""]] -> w730 mode=indexing
            i -> [w764]
            w768 = 0 ("인덱스 (행)")
            n286 = Index Array(array=w770) -> (element=w769:string)  [unwired: 1 in]
            n287 = Multiply(x=w764, y=3) -> (x*y=w762:i32)
            n288 = Replace Array Subset(array=string[][] [["", "", ""], ["", "", ""], ["", "", ""], ["", "", ""], ["", "", ""], ["", "", ""], ["", "", ""], ["", "", ""]], new element=w769, index (row)=w768, index (col)=w768) -> (w767:string[][])
            n289 = Insert Into Array(array=w766, index (col)=w762, new element=w767) -> (w765:string[][])  [unwired: 1 in]
          }
          n290 = call-poly "Table Initialize.vi"("Table Ref"=w725, "Value"=w715, "에러 입력"=w741) -> ("에러 출력"=w728:errorcluster)  [unwired: 6 in, 2 out]
          n291 = call "STD Cal Data_etc.vi"("error in"=w728, "Func_ext"=w747) -> ("error out"=w737:errorcluster, "Data Out"=w722:string[][], "Func_ext Out"=w721:string)  [unwired: 5 in, 2 out]
          n292 = Index Array(array=w755) -> (element=w745:refnum<vi>)  [unwired: 1 in]
          n293 = Index Array(array=w759) -> (element=w749:refnum<vi>)  [unwired: 1 in]
          n294 = call "Get Spec.vi"("NumRows"=u32 28, "Spec in"=w723, "Spec Ref."=w745, "error in"=w737, "Condition in"=w715, "Resolution in"=w722, "Func_ext"=w721) -> ("error out"=w744:errorcluster, "Data Out"=w726:string[][], "Func_ext Out"=w743:string)  [unwired: 2 out]
          n295 = call "Match_CMC.vi"("CMC IN"=w750, "error in"=w744, "Condition IN"=w726, "Func_ext"=w743) -> ("error out"=w739:errorcluster, "Func_ext out"=w736:string)  [unwired: 4 in, 2 out]
          n296 = property class="MCListbox (엄격한)"(reference=w749, error in=w739, "TopLeft"=cluster{"Row":u32, "Column":u32} {"Row"=0, "Column"=0} ("왼쪽 위에 보이는 셀"), "Value"=-1 ("값"), "ItemNames"=w715) -> (error out=w719:errorcluster)  [unwired: 1 out]
          n297 = Index Array(array=w757) -> (element=w727:refnum<vi>)  [unwired: 1 in]
          n298 = call "Variables Data IO.vi"("Select"=Cmd_Var_Data_IO."Result_Temp", "error in"=w719, "Data In"=w730, "Func_ext"=w736) -> ("error out"=w734:errorcluster, "Func_ext Out"=w733:string)  [unwired: 5 in, 1 out]
          n299 = call "Variables Data IO.vi"("Select"=Cmd_Var_Data_IO."Result", "error in"=w734, "Data In"=w729, "Func_ext"=w733) -> ("error out"=w718:errorcluster)  [unwired: 5 in, 2 out]
          n300 = property class="Tbl (엄격한)"(reference=w727, error in=w718, "Value"=w753) -> (error out=w717:errorcluster)  [unwired: 1 out]
          n301 = Index Array(array=w754) -> (element=w738:refnum<vi>)  [unwired: 1 in]
          n302 = property class="Str"(reference=w738, error in=w717, "Value"=w720) -> (error out=w716:errorcluster)  [unwired: 1 out]
          n303 = for {
            tunnel: w756 -> [w771] mode=indexing
            shift-right: [w772] -> w752
            shift-left: w716 -> [w773]
            n304 = call-poly "Table Initialize.vi"("Table Ref"=w771, "에러 입력"=w773) -> ("에러 출력"=w772:errorcluster)  [unwired: 7 in, 2 out]
          }
        }
      }
    }
    frame "Pressure_1" {
      w855 = 0 ("인덱스 (행)")
      n305 = Unbundle By Name(w859) -> ("Initialize 2.문자열"=w798:refnum<vi>[], "Initialize 2.콤보박스"=w806:refnum<vi>[], "Initialize 2.테이블"=w821:refnum<vi>[], "Initialize 1.Spec"=w846:refnum<vi>[], "Initialize 1.Condition"=w819:refnum<vi>[], "Initialize 1.Resolution"=w856:refnum<vi>[])
      n306 = call "Get Calproc.vi"("제목"=w824, "에러 입력"=w858, "Func_ext"=w840) -> ("에러 출력"=w857:errorcluster, "Condition"=w823:string[][], "Func_ext Out"=w825:string, "클러스터"=w838:T5)  [unwired: 5 in]
      n307 = Unbundle By Name(w838) -> ("Resolution"=w844:string[][], "Spec"=w833:string[][], "CMC"=w841:string[][], "Condition"=w822:string[][], "NumRows"=w817:u32)
      n308 = call "Variables Data IO.vi"("Select"=Cmd_Var_Data_IO."Condition Default", "error in"=w857, "Data In"=w823, "Func_ext"=w825) -> ("error out"=w826:errorcluster, "Func_ext Out"=w827:string)  [unwired: 5 in, 1 out]
      n309 = Index Array(array=w856) -> (element=w830:refnum<vi>)  [unwired: 1 in]
      n310 = call "Create Resolution.vi"("행의 개수"=w817, "Table Ref"=w830, "에러 입력(에러 없음)"=w826, "Resolution"=w844, "Func_ext"=w827) -> ("에러 출력"=w829:errorcluster, "Resolution Out"=w832:string[][], "Func_ext 출력"=w828:string)  [unwired: 4 in]
      n311 = Index Array(array=w819) -> (element=w839:refnum<vi>)  [unwired: 1 in]
      n312 = call "STD Cal Data_etc.vi"("error in"=w829, "Func_ext"=w828) -> ("error out"=w850:errorcluster, "Data Out"=w803:string[][], "Func_ext Out"=w848:string, "Data Out 2"=w813:string[])  [unwired: 5 in, 1 out]
      n313 = Index Array(array=w846) -> (element=w854:refnum<vi>)  [unwired: 1 in]
      n314 = call-poly "Table Initialize.vi"("행의 개수"=w817, "Table Ref"=w839, "Value"=w803, "에러 입력"=w850) -> ("에러 출력"=w849:errorcluster, "Bottom"=w818:i32)  [unwired: 5 in, 1 out]
      n315 = call "Variables Data IO.vi"("Select"=Cmd_Var_Data_IO."Condition", "error in"=w849, "Data In"=w803, "Func_ext"=w848) -> ("error out"=w842:errorcluster, "Func_ext Out"=w831:string)  [unwired: 5 in, 1 out]
      n316 = Index Array(array=w821) -> (element=w820:refnum<vi>)  [unwired: 1 in]
      n317 = call "Get Spec.vi"("NumRows"=w817, "Spec in"=w833, "Spec Ref."=w854, "error in"=w842, "Condition in"=w803, "Resolution in"=w832, "Func_ext"=w831) -> ("error out"=w853:errorcluster, "Data Out"=w843:string[][], "Func_ext Out"=w852:string)  [unwired: 2 out]
      n318 = call "Match_CMC.vi"("CMC IN"=w841, "error in"=w853, "Condition IN"=w843, "Func_ext"=w852) -> ("error out"=w815:errorcluster, "Func_ext out"=w812:string)  [unwired: 4 in, 2 out]
      n319 = call "Variables Data IO.vi"("Select"=Cmd_Var_Data_IO."Condition_Temp", "error in"=w815, "Func_ext"=w812) -> ("error out"=w811:errorcluster, "Data Out"=w794:string[][], "Func_ext Out"=w816:string)  [unwired: 6 in]
      n320 = Empty Array?(array=w794) -> (empty?=w793:bool)
      n321 = case shown="거짓" w793 {
        tunnel: w820 -> [w872 w874]
        tunnel: w818 -> [w871 _]
        tunnel: w817 -> [w870 _]
        tunnel: w813 -> [w861 _]
        tunnel: w811 -> [w869 w876]
        tunnel: w794 -> [w867 _]
        tunnel: [w865 w875] -> w805
        frame False {
          n322 = call-poly "Remove Empty Array.vi"("조건"=enum16{"행", "열", "행,열"}."열", "error in (no error)"=w869, "Data in"=w867) -> ("error out"=w868:errorcluster, "Data out"=w864:string[][])  [unwired: 7 in]
          n323 = call-poly "Cell Spacing.vi"("Row Header in"=w861, "error in"=w868, "Data in"=w864, "테이블 참조 in"=w872) -> ("error out"=w863:errorcluster, "테이블 참조 Out"=w862:refnum<vi>)  [unwired: 5 in, 1 out]
          n324 = property on="std set" class="Tbl"(reference=w862, error in=w863, "Visible"=TRUE ("보이기"), "Top"=w871, "Number of Rows"=w870) -> (error out=w865:errorcluster)  [unwired: 1 out]
        }
        frame True {
          n325 = property on="std set" class="Tbl (엄격한)"(reference=w874, error in=w876, "Visible"=FALSE ("보이기")) -> (error out=w875:errorcluster)  [unwired: 1 out]
        }
      }
      n326 = Delete From Array(array=w806) -> (deleted portion=w804:refnum<vi>, array with subset deleted=w802:refnum<vi>[])  [unwired: 2 in]
      n327 = property on="교정방법" class="CmbBox"(reference=w804, error in=w805) -> (error out=w797:errorcluster, "Value"=w845:string)  [unwired: 1 out]
      n328 = call "Pressure Cal Point.vi"("Condition"=w822, "교정방법"=w845) -> ("배열"=w834:string[][], "단위"=w808:string, "최소용량"=w809:string, "최대용량"=w810:string)  [unwired: 6 in]
      n329 = Index Array(array=w832, index (row) #1=w855, index (col) #1=w855) -> (element #1=w801:string, element #2=w800:string)  [unwired: 2 in]
      n330 = Build Array(w801, w800) -> (w799:string[])
      n331 = Build Array(w810, w809, w808) -> (w807:string[])
      n332 = call-poly "String Contents.vi"("문자 배열"=w807, "참조 배열"=w798, "에러 입력"=w797) -> ("에러 출력"=w796:errorcluster)  [unwired: 7 in, 1 out]
      n333 = call-poly "String Contents.vi"("문자 배열"=w799, "참조 배열"=w802, "에러 입력"=w796) -> ("에러 출력"=w795:errorcluster)  [unwired: 7 in, 1 out]
      n334 = call "Certi Recall.vi"("Value"=w834, "큐 입력"=w836, "NumRows"=w817, "입력 클러스터"=w835, "에러 입력"=w795, "Text in"=w801, "Func_ext in"=w816) -> ("에러 출력"=w837:errorcluster)  [unwired: 3 in, 1 out]
    }
    frame "Pressure_2" {
      n335 = Unbundle By Name(w950) -> ("Initialize 2.문자열"=w883:refnum<vi>[], "Initialize 1.Spec"=w920:refnum<vi>[], "Initialize 2.테이블"=w919:refnum<vi>[], "Initialize 1.Condition"=w941:refnum<vi>[], "Initialize 1.Resolution"=w948:refnum<vi>[], "Initialize 2.디지털(DBL)"=w901:refnum<vi>[], "Initialize 2.콤보박스"=w895:refnum<vi>[])
      n336 = call "Get Calproc.vi"("제목"=w921, "에러 입력"=w949, "Func_ext"=w937) -> ("에러 출력"=w892:errorcluster, "Condition"=w879:string[][], "Func_ext Out"=w887:string, "클러스터"=w931:T5)  [unwired: 5 in]
      n337 = Unbundle By Name(w931) -> ("Spec"=w927:string[][], "CMC"=w938:string[][], "NumRows"=w913:u32)
      n338 = for {
        tunnel: w895 -> [w968] mode=indexing
        shift-right: [w967] -> w891
        shift-left: w892 -> [w966]
        tunnel: [w965] -> w894 mode=indexing
        n339 = property class="CmbBox"(reference=w968, error in=w966) -> (error out=w967:errorcluster, "Value"=w965:string)  [unwired: 1 out]
      }
      n340 = for {
        tunnel: w901 -> [w972] mode=indexing
        shift-right: [w971] -> w889
        shift-left: w891 -> [w970]
        tunnel: [w969] -> w900 mode=indexing
        n341 = property class="DigNum (엄격한)"(reference=w972, error in=w970) -> (error out=w971:errorcluster, "Value"=w969:dbl)  [unwired: 1 out]
      }
      n342 = Index Array(array=w894) -> (element #1=w893:string, element #2=w890:string)  [unwired: 2 in]
      n343 = Index Array(array=w900) -> (element #1=w898:dbl, element #2=w899:dbl, element #3=w897:dbl)  [unwired: 3 in]
      n344 = case shown="\"mV/V\"" w893 {
        selector: w893 -> [w988 w997 w1008 w1014]
        tunnel: ["0.00001" "0.0001" "0.0001" "0.0001"] -> w903
        tunnel: w898 -> [w989 w998 w1004 _]
        tunnel: w899 -> [w986 w995 w1001 _]
        tunnel: w897 -> [w985 w994 w1003 _]
        tunnel: [w988 w997 w1008 w1014] -> w935
        tunnel: [w987 w996 w1007 ""] -> w934
        tunnel: [w984 w993 w1006 ""] -> w933
        tunnel: [w983 w992 w1005 ""] -> w932
        tunnel: w879 -> [w982 w991 w1000 w1010]
        tunnel: [w982 w991 w1000 w1010] -> w896
        frame "V" {
          n345 = Number To Fractional String(number=w989) -> (F-format string=w987:string)  [unwired: 3 in]
          n346 = Number To Fractional String(number=w986) -> (F-format string=w984:string)  [unwired: 3 in]
          n347 = Number To Fractional String(number=w985) -> (F-format string=w983:string)  [unwired: 3 in]
        }
        frame "mA" {
          n348 = Number To Fractional String(number=w998) -> (F-format string=w996:string)  [unwired: 3 in]
          n349 = Number To Fractional String(number=w995) -> (F-format string=w993:string)  [unwired: 3 in]
          n350 = Number To Fractional String(number=w994) -> (F-format string=w992:string)  [unwired: 3 in]
        }
        frame "mV/V" {
          n351 = Multiply(x=w1001, y=w1003) -> (x*y=w1002:dbl)
          n352 = Number To Fractional String(number=w1004) -> (F-format string=w1007:string)  [unwired: 3 in]
          n353 = Number To Fractional String(number=w1002) -> (F-format string=w1006:string)  [unwired: 3 in]
          n354 = Number To Fractional String(number=w1003) -> (F-format string=w1005:string)  [unwired: 3 in]
        }
        frame Default {
        }
      }
      n355 = call "Pressure Cal Point.vi"("Condition"=w879, "교정방법"=w890) -> ("배열"=w880:string[][], "단위"=w904:string, "최소용량"=w905:string, "최대용량"=w906:string)  [unwired: 6 in]
      n356 = for {
        tunnel: w903 -> [w981]
        tunnel: w935 -> [w973]
        tunnel: [w980] -> w936 mode=indexing
        tunnel: w896 -> [w978] mode=indexing
        tunnel: [w977] -> w878 mode=indexing
        tunnel: w934 -> [w976]
        tunnel: w933 -> [w975]
        tunnel: w932 -> [w974]
        n357 = Insert Into Array(array=w978, new element #1=w976, new element #2=w975, new element #3=w974, new element #4=w973) -> (w977:string[])  [unwired: 1 in]
        n358 = Build Array("Digital" ("원소"), w981, w973) -> (w980:string[])
      }
      n359 = Build Array(w906, w905, w904, w903) -> (w902:string[])
      n360 = Index Array(array=w948) -> (element=w924:refnum<vi>)  [unwired: 1 in]
      n361 = call "Variables Data IO.vi"("Select"=Cmd_Var_Data_IO."Condition Default", "error in"=w889, "Data In"=w878, "Func_ext"=w887) -> ("error out"=w888:errorcluster, "Func_ext Out"=w886:string)  [unwired: 5 in, 1 out]
      n362 = Index Array(array=w941) -> (element=w918:refnum<vi>)  [unwired: 1 in]
      n363 = call "Create Resolution.vi"("행의 개수"=w913, "Table Ref"=w924, "에러 입력(에러 없음)"=w888, "Resolution"=w936, "Func_ext"=w886) -> ("에러 출력"=w923:errorcluster, "Resolution Out"=w926:string[][], "Func_ext 출력"=w922:string)  [unwired: 4 in]
      n364 = call "STD Cal Data_etc.vi"("error in"=w923, "Func_ext"=w922) -> ("error out"=w943:errorcluster, "Data Out"=w877:string[][], "Func_ext Out"=w909:string, "Data Out 2"=w912:string[])  [unwired: 5 in, 1 out]
      n365 = call-poly "Table Initialize.vi"("행의 개수"=w913, "Table Ref"=w918, "Value"=w877, "에러 입력"=w943) -> ("에러 출력"=w911:errorcluster, "Bottom"=w914:i32)  [unwired: 5 in, 1 out]
      n366 = Index Array(array=w919) -> (element=w915:refnum<vi>)  [unwired: 1 in]
      n367 = call "Variables Data IO.vi"("Select"=Cmd_Var_Data_IO."Condition_Temp", "error in"=w911, "Func_ext"=w909) -> ("error out"=w910:errorcluster, "Data Out"=w882:string[][], "Func_ext Out"=w908:string)  [unwired: 6 in]
      n368 = Empty Array?(array=w882) -> (empty?=w881:bool)
      n369 = case shown="거짓" w881 {
        tunnel: [w958 w962] -> w916
        tunnel: w915 -> [w957 w963]
        tunnel: w914 -> [w956 _]
        tunnel: w913 -> [w955 _]
        tunnel: w912 -> [w954 _]
        tunnel: w910 -> [w953 w964]
        tunnel: w882 -> [w952 _]
        frame False {
          n370 = call-poly "Cell Spacing.vi"("Row Header in"=w954, "error in"=w953, "Data in"=w952, "테이블 참조 in"=w957) -> ("error out"=w960:errorcluster, "테이블 참조 Out"=w959:refnum<vi>)  [unwired: 5 in, 1 out]
          n371 = property on="std set" class="Tbl"(reference=w959, error in=w960, "Top"=w956, "Number of Rows"=w955, "Visible"=TRUE ("보이기")) -> (error out=w958:errorcluster)  [unwired: 1 out]
        }
        frame True {
          n372 = property on="std set" class="Tbl (엄격한)"(reference=w963, error in=w964, "Visible"=FALSE ("보이기")) -> (error out=w962:errorcluster)  [unwired: 1 out]
        }
      }
      n373 = Index Array(array=w920) -> (element=w947:refnum<vi>)  [unwired: 1 in]
      n374 = call "Variables Data IO.vi"("Select"=Cmd_Var_Data_IO."Condition", "error in"=w916, "Data In"=w877, "Func_ext"=w908) -> ("error out"=w939:errorcluster, "Func_ext Out"=w925:string)  [unwired: 5 in, 1 out]
      n375 = call "Get Spec.vi"("NumRows"=w913, "Spec in"=w927, "Spec Ref."=w947, "error in"=w939, "Condition in"=w877, "Resolution in"=w926, "Func_ext"=w925) -> ("error out"=w946:errorcluster, "Data Out"=w940:string[][], "Func_ext Out"=w945:string)  [unwired: 2 out]
      n376 = call "Match_CMC.vi"("CMC IN"=w938, "error in"=w946, "Condition IN"=w940, "Func_ext"=w945) -> ("error out"=w885:errorcluster, "Func_ext out"=w928:string)  [unwired: 4 in, 2 out]
      n377 = call-poly "String Contents.vi"("문자 배열"=w902, "참조 배열"=w883, "에러 입력"=w885) -> ("에러 출력"=w884:errorcluster)  [unwired: 7 in, 1 out]
      n378 = call "Certi Recall.vi"("Value"=w880, "큐 입력"=w930, "NumRows"=w913, "입력 클러스터"=w929, "에러 입력"=w884, "Func_ext in"=w928) -> ("에러 출력"=w917:errorcluster)  [unwired: 4 in, 1 out]
    }
    frame "Pressure_3" {
      w1087 = 0 ("인덱스 (행)")
      n379 = Unbundle By Name(w1091) -> ("Initialize 1.Spec"=w1080:refnum<vi>[], "Initialize 1.Condition"=w1074:refnum<vi>[], "Initialize 2.문자열"=w1036:refnum<vi>[], "Initialize 2.콤보박스"=w1040:refnum<vi>[], "Initialize 1.Resolution"=w1088:refnum<vi>[])
      n380 = call "Get Calproc.vi"("제목"=w1054, "에러 입력"=w1090, "Func_ext"=w1075) -> ("에러 출력"=w1089:errorcluster, "Condition"=w1049:string[][], "Func_ext Out"=w1058:string, "클러스터"=w1067:T5)  [unwired: 5 in]
      n381 = Unbundle By Name(w1067) -> ("Resolution"=w1078:string[][], "Spec"=w1062:string[][], "CMC"=w1076:string[][], "NumRows"=w1053:u32)
      n382 = call "Variables Data IO.vi"("Select"=Cmd_Var_Data_IO."Condition Default", "error in"=w1089, "Data In"=w1049, "Func_ext"=w1058) -> ("error out"=w1056:errorcluster, "Func_ext Out"=w1057:string)  [unwired: 5 in, 1 out]
      n383 = Index Array(array=w1088) -> (element=w1059:refnum<vi>)  [unwired: 1 in]
      n384 = call "Create Resolution.vi"("행의 개수"=w1053, "Table Ref"=w1059, "에러 입력(에러 없음)"=w1056, "Resolution"=w1078, "Func_ext"=w1057) -> ("에러 출력"=w1033:errorcluster, "Resolution Out"=w1061:string[][], "Func_ext 출력"=w1055:string)  [unwired: 4 in]
      n385 = Delete From Array(array=w1040, length=2 ("길이")) -> (deleted portion=w1034:refnum<vi>[], array with subset deleted=w1035:refnum<vi>[])  [unwired: 1 in]
      n386 = Index Array(array=w1061, index (row) #1=w1087, index (col) #1=w1087) -> (element #1=w1042:string, element #2=w1046:string)  [unwired: 2 in]
      n387 = Build Array(w1042, w1046) -> (w1045:string[])
      n388 = call-poly "String Contents.vi"("문자 배열"=w1045, "참조 배열"=w1034, "에러 입력"=w1033) -> ("에러 출력"=w1032:errorcluster)  [unwired: 7 in, 1 out]
      n389 = Index Array(array=w1035) -> (element #1=w1038:refnum<vi>, element #2=w1039:refnum<vi>)  [unwired: 2 in]
      n390 = Delete From Array(array=w1036) -> (deleted portion=w1028:refnum<vi>, array with subset deleted=w1044:refnum<vi>[])  [unwired: 2 in]
      n391 = property on="유체" class="CmbBox"(reference=w1039, error in=w1032) -> (error out=w1018:errorcluster, "Value"=w1023:string)  [unwired: 1 out]
      n392 = Equal?(x=w1023, y="담수") -> (x = y?=w1027:bool)
      n393 = Select(t=T4."Enabled" ("비활성화"), s=w1027, f=T4."Disabled and Grayed Out" ("비활성화")) -> (s? t:f=w1024:T4)
      n394 = property on="기준온도" class="Str"(reference=w1028, error in=w1018, "DisabledEnum"=w1024) -> (error out=w1017:errorcluster, "Value"=w1022:string)  [unwired: 1 out]
      n395 = Build Array(w1022, w1023) -> (w1021:string[])
      n396 = property on="교정방법" class="CmbBox"(reference=w1038, error in=w1017) -> (error out=w1016:errorcluster, "Value"=w1079:string)  [unwired: 1 out]
      n397 = Build Array(w1021) -> (w1019:string[][])
      n398 = call "STD Cal Data_etc.vi"("error in"=w1016, "Data in"=w1019, "Func_ext"=w1055) -> ("error out"=w1031:errorcluster, "Data Out"=w1048:string[][], "Func_ext Out"=w1082:string)  [unwired: 4 in, 2 out]
      n399 = Index Array(array=w1048, index (col)=4 ("비활성화된 인덱스 (열)")) -> (element=w1072:string[])  [unwired: 1 in]
      n400 = call "Variables Data IO.vi"("Select"=Cmd_Var_Data_IO."Condition", "error in"=w1031, "Data In"=w1048, "Func_ext"=w1082) -> ("error out"=w1020:errorcluster, "Func_ext Out"=w1060:string)  [unwired: 5 in, 1 out]
      n401 = Fract/Exp String To Number(string=w1072) -> (number=w1071:dbl[])  [unwired: 3 in, 1 out]
      n402 = Array Max & Min(array=w1071) -> (max value=w1070:dbl)  [unwired: 3 out]
      n403 = call "Number Format.vi"("입력값"=w1046) -> ("정밀도(단위적용)"=w1069:i32)  [unwired: 10 in]
      n404 = Number To Fractional String(number=w1070, precision (6)=w1069) -> (F-format string=w1050:string)  [unwired: 2 in]
      n405 = call "Pressure Cal Point.vi"("Condition"=w1049, "교정방법"=w1079) -> ("배열"=w1065:string[][], "최대용량"=w1052:string)  [unwired: 6 in, 2 out]
      n406 = Build Array(w1050, w1052) -> (w1051:string[])
      n407 = call-poly "String Contents.vi"("문자 배열"=w1051, "참조 배열"=w1044, "에러 입력"=w1020) -> ("에러 출력"=w1029:errorcluster)  [unwired: 7 in, 1 out]
      n408 = Index Array(array=w1074) -> (element=w1068:refnum<vi>)  [unwired: 1 in]
      n409 = call-poly "Table Initialize.vi"("행의 개수"=w1053, "Table Ref"=w1068, "Value"=w1048, "에러 입력"=w1029) -> ("에러 출력"=w1030:errorcluster)  [unwired: 5 in, 2 out]
      n410 = Index Array(array=w1080) -> (element=w1086:refnum<vi>)  [unwired: 1 in]
      n411 = call "Get Spec.vi"("NumRows"=w1053, "Spec in"=w1062, "Spec Ref."=w1086, "error in"=w1030, "Condition in"=w1048, "Resolution in"=w1061, "Func_ext"=w1060) -> ("error out"=w1085:errorcluster, "Data Out"=w1077:string[][], "Func_ext Out"=w1084:string)  [unwired: 2 out]
      n412 = call "Match_CMC.vi"("CMC IN"=w1076, "error in"=w1085, "Condition IN"=w1077, "Func_ext"=w1084) -> ("error out"=w1037:errorcluster, "Func_ext out"=w1047:string)  [unwired: 4 in, 2 out]
      n413 = call "Certi Recall.vi"("Value"=w1065, "큐 입력"=w1066, "NumRows"=w1053, "입력 클러스터"=w1064, "에러 입력"=w1037, "Text in"=w1042, "Func_ext in"=w1047) -> ("에러 출력"=w1063:errorcluster)  [unwired: 3 in, 1 out]
    }
    frame "Pressure_4" {
      n414 = Unbundle By Name(w1141) -> ("Initialize 2.테이블"=w1104:refnum<vi>[], "Initialize 2.콤보박스"=w1117:refnum<vi>[], "Initialize 2.문자열"=w1116:refnum<vi>[], "Initialize 1.Spec"=w1120:refnum<vi>[], "Initialize 1.Resolution"=w1139:refnum<vi>[], "Initialize 1.Condition"=w1124:refnum<vi>[])
      n415 = call "Get Calproc.vi"("제목"=w1125, "에러 입력"=w1140, "Func_ext"=w1133) -> ("에러 출력"=w1099:errorcluster, "Condition"=w1094:string[][], "Func_ext Out"=w1100:string, "클러스터"=w1131:T5)  [unwired: 5 in]
      n416 = Unbundle By Name(w1131) -> ("Resolution"=w1112:string[][], "Spec"=w1127:string[][], "CMC"=w1134:string[][], "NumRows"=w1101:u32)
      n417 = call "Variables Data IO.vi"("Select"=Cmd_Var_Data_IO."Condition Default", "error in"=w1099, "Data In"=w1094, "Func_ext"=w1100) -> ("error out"=w1098:errorcluster, "Func_ext Out"=w1097:string)  [unwired: 5 in, 1 out]
      n418 = for {
        tunnel: w1094 -> [w1145] mode=indexing
        tunnel: [w1142] -> w1095 mode=indexing
        n419 = Insert Into Array(array=w1145, index=1 ("인덱스"), new element="" ("새 원소/부분배열")) -> (w1142:string[])
      }
      n420 = Index Array(array=w1124) -> (element=w1132:refnum<vi>)  [unwired: 1 in]
      n421 = call "Variables Data IO.vi"("Select"=Cmd_Var_Data_IO."Condition", "error in"=w1098, "Data In"=w1095, "Func_ext"=w1097) -> ("Func_ext Out"=w1096:string)  [unwired: 5 in, 2 out]
      n422 = call-poly "Table Initialize.vi"("행의 개수"=w1101, "Table Ref"=w1132, "Value"=w1095, "에러 입력"=w1098) -> ("에러 출력"=w1123:errorcluster)  [unwired: 5 in, 2 out]
      n423 = Index Array(array=w1139) -> (element=w1126:refnum<vi>)  [unwired: 1 in]
      n424 = call "Create Resolution.vi"("행의 개수"=w1101, "Table Ref"=w1126, "에러 입력(에러 없음)"=w1123, "Resolution"=w1112, "Func_ext"=w1096) -> ("에러 출력"=w1121:errorcluster, "Resolution Out"=w1113:string[][], "Func_ext 출력"=w1122:string)  [unwired: 4 in]
      n425 = Index Array(array=w1120) -> (element=w1138:refnum<vi>)  [unwired: 1 in]
      n426 = call "Get Spec.vi"("NumRows"=w1101, "Spec in"=w1127, "Spec Ref."=w1138, "error in"=w1121, "Condition in"=w1095, "Resolution in"=w1113, "Func_ext"=w1122) -> ("error out"=w1118:errorcluster, "Data Out"=w1135:string[][], "Func_ext Out"=w1119:string)  [unwired: 2 out]
      n427 = call "Match_CMC.vi"("CMC IN"=w1134, "error in"=w1118, "Condition IN"=w1135, "Func_ext"=w1119) -> ("error out"=w1114:errorcluster, "Func_ext out"=w1093:string)  [unwired: 4 in, 2 out]
      n428 = call "Extract String.vi"("Resolution"=w1112, "Condition"=w1094) -> ("배열 1"=w1109:string[], "배열 2"=w1111:string[])  [unwired: 7 in, 1 out]
      n429 = Build Array (concatenate)(w1117, w1116) -> (w1115:refnum<vi>[])
      n430 = Index Array(array=w1111, index=2 ("인덱스")) -> (element=w1108:string)
      n431 = Insert Into Array(array=w1109, new element=w1108) -> (w1107:string[])  [unwired: 1 in]
      n432 = call-poly "String Contents.vi"("문자 배열"=w1107, "참조 배열"=w1115, "에러 입력"=w1114) -> ("에러 출력"=w1105:errorcluster)  [unwired: 7 in, 1 out]
      n433 = Index Array(array=w1104) -> (element=w1103:refnum<vi>)  [unwired: 1 in]
      n434 = call-poly "Table Initialize.vi"("행의 개수"=w1101, "Table Ref"=w1103, "에러 입력"=w1105) -> ("에러 출력"=w1102:errorcluster)  [unwired: 6 in, 2 out]
      n435 = call "STD Cal Data_etc.vi"("error in"=w1102, "Func_ext"=w1093) -> ("error out"=w1106:errorcluster, "Func_ext Out"=w1092:string)  [unwired: 5 in, 3 out]
      n436 = call "Certi Recall.vi"("Value"=w1095, "큐 입력"=w1130, "NumRows"=w1101, "입력 클러스터"=w1129, "에러 입력"=w1106, "Func_ext in"=w1092) -> ("에러 출력"=w1128:errorcluster)  [unwired: 4 in, 1 out]
    }
    frame "Torque_1" {
      w1195 = 1 ("인덱스 (행)")
      w1191 = 0 ("인덱스 (행)")
      n437 = Unbundle By Name(w1206) -> ("Initialize 2.콤보박스"=w1146:refnum<vi>[], "Initialize 2.문자열"=w1157:refnum<vi>[], "Initialize 2.테이블"=w1167:refnum<vi>[], "Initialize 1.Condition"=w1192:refnum<vi>[], "Initialize 1.Spec"=w1156:refnum<vi>[])
      n438 = call "Get Calproc.vi"("제목"=w1163, "에러 입력"=w1205, "Func_ext"=w1194) -> ("에러 출력"=w1204:errorcluster, "Condition"=w1162:string[][], "Func_ext Out"=w1199:string, "클러스터"=w1175:T5)  [unwired: 5 in]
      n439 = Unbundle By Name(w1175) -> ("Resolution"=w1153:string[][], "Spec"=w1155:string[][], "CMC"=w1154:string[][], "NumRows"=w1166:u32, "Resolution"=w1152:string[][])
      n440 = call "Variables Data IO.vi"("Select"=Cmd_Var_Data_IO."Condition Default", "error in"=w1204, "Data In"=w1162, "Func_ext"=w1199) -> ("error out"=w1190:errorcluster, "Func_ext Out"=w1187:string)  [unwired: 5 in, 1 out]
      n441 = call "Create Resolution.vi"("에러 입력(에러 없음)"=w1190, "Resolution"=w1153, "Func_ext"=w1187) -> ("에러 출력"=w1189:errorcluster, "Resolution Out"=w1165:string[][], "Func_ext 출력"=w1186:string)  [unwired: 6 in]
      n442 = Index Array(array=w1156) -> (element=w1201:refnum<vi>)  [unwired: 1 in]
      n443 = call "STD Cal Data_etc.vi"("error in"=w1189, "Func_ext"=w1186) -> ("error out"=w1188:errorcluster, "Data Out"=w1151:string[][], "Func_ext Out"=w1185:string)  [unwired: 5 in, 2 out]
      n444 = Index Array(array=w1192) -> (element=w1177:refnum<vi>)  [unwired: 1 in]
      n445 = call "Variables Data IO.vi"("Select"=Cmd_Var_Data_IO."Condition", "error in"=w1188, "Data In"=w1151, "Func_ext"=w1185) -> ("error out"=w1169:errorcluster, "Func_ext Out"=w1164:string)  [unwired: 5 in, 1 out]
      n446 = call "Get Spec.vi"("NumRows"=w1166, "Spec in"=w1155, "Spec Ref."=w1201, "error in"=w1169, "Condition in"=w1151, "Resolution in"=w1165, "Func_ext"=w1164) -> ("error out"=w1197:errorcluster, "Data Out"=w1193:string[][], "Func_ext Out"=w1200:string)  [unwired: 2 out]
      n447 = call "Match_CMC.vi"("CMC IN"=w1154, "error in"=w1197, "Condition IN"=w1193, "Func_ext"=w1200) -> ("error out"=w1170:errorcluster, "Func_ext out"=w1183:string)  [unwired: 4 in, 2 out]
      n448 = Index Array(array=w1167) -> (element=w1181:refnum<vi>)  [unwired: 1 in]
      n449 = call-poly "Table Initialize.vi"("행의 개수"=w1166, "Table Ref"=w1177, "Value"=w1151) -> ("Bottom"=w1176:i32)  [unwired: 6 in, 2 out]
      n450 = call "Variables Data IO.vi"("Select"=Cmd_Var_Data_IO."STD2", "error in"=w1170, "Func_ext"=w1183) -> ("error out"=w1179:errorcluster, "Data Out"=w1182:string[][], "Func_ext Out"=w1171:string)  [unwired: 6 in]
      n451 = Index Array(array=w1151, index (row) #1=w1195, index (col) #1=0 ("비활성화된 인덱스 (열)"), index (row) #2=w1195, index (col) #2=w1195) -> (element #1=w1161:string, element #2=w1160:string)
      n452 = Index Array(array=w1152, index (row) #1=w1191, index (col) #1=1 ("비활성화된 인덱스 (열)"), index (row) #2=w1191, index (col) #2=w1191) -> (element #1=w1148:string, element #2=w1159:string)
      n453 = call-poly "Cell Spacing.vi"("error in"=w1179, "Data in"=w1182, "테이블 참조 in"=w1181) -> ("error out"=w1178:errorcluster, "테이블 참조 Out"=w1180:refnum<vi>)  [unwired: 6 in, 1 out]
      n454 = Build Array(w1161, w1160, w1159) -> (w1158:string[])
      n455 = Build Array(w1148) -> (w1147:string[])
      n456 = property on="Condition 2" class="Tbl"(reference=w1180, error in=w1178, "Top"=w1176, "Number of Rows"=w1166) -> (error out=w1168:errorcluster)  [unwired: 1 out]
      n457 = call-poly "String Contents.vi"("문자 배열"=w1158, "참조 배열"=w1157, "에러 입력"=w1168) -> ("에러 출력"=w1150:errorcluster)  [unwired: 7 in, 1 out]
      n458 = call-poly "String Contents.vi"("문자 배열"=w1147, "참조 배열"=w1146, "에러 입력"=w1150) -> ("에러 출력"=w1149:errorcluster)  [unwired: 7 in, 1 out]
      n459 = call "Certi Recall.vi"("큐 입력"=w1173, "NumRows"=w1166, "입력 클러스터"=w1172, "에러 입력"=w1149, "Func_ext in"=w1171) -> ("에러 출력"=w1174:errorcluster)  [unwired: 5 in, 1 out]
    }
    frame "Torque_2" {
      w1235 = 0 ("인덱스 (행)")
      w1261 = 1 ("인덱스 (행)")
      n460 = Unbundle By Name(w1272) -> ("Initialize 2.콤보박스"=w1237:refnum<vi>[], "Initialize 2.문자열"=w1247:refnum<vi>[], "Initialize 1.Condition"=w1265:refnum<vi>[], "Initialize 1.Spec"=w1251:refnum<vi>[])
      n461 = call "Get Calproc.vi"("제목"=w1253, "에러 입력"=w1271, "Func_ext"=w1260) -> ("에러 출력"=w1270:errorcluster, "Condition"=w1219:string[][], "Func_ext Out"=w1266:string, "클러스터"=w1252:T5)  [unwired: 5 in]
      n462 = Unbundle By Name(w1252) -> ("Resolution"=w1242:string[][], "Spec"=w1254:string[][], "CMC"=w1226:string[][], "NumRows"=w1255:u32)
      n463 = call "Variables Data IO.vi"("Select"=Cmd_Var_Data_IO."Condition Default", "error in"=w1270, "Data In"=w1219, "Func_ext"=w1266) -> ("error out"=w1232:errorcluster, "Func_ext Out"=w1233:string)  [unwired: 5 in, 1 out]
      n464 = call "Create Resolution.vi"("에러 입력(에러 없음)"=w1232, "Resolution"=w1242, "Func_ext"=w1233) -> ("에러 출력"=w1230:errorcluster, "Func_ext 출력"=w1231:string)  [unwired: 6 in, 1 out]
      n465 = call "STD Cal Data_etc.vi"("error in"=w1230, "Func_ext"=w1231) -> ("error out"=w1229:errorcluster, "Func_ext Out"=w1215:string, "Data Out 2"=w1214:string[])  [unwired: 5 in, 2 out]
      n466 = Index Array(array=w1251) -> (element=w1268:refnum<vi>)  [unwired: 1 in]
      n467 = Delete From Array(array=w1214) -> (deleted portion=w1212:string, array with subset deleted=w1213:string[])  [unwired: 2 in]
      n468 = Index Array(array=w1265) -> (element=w1259:refnum<vi>)  [unwired: 1 in]
      n469 = for {
        tunnel: w1219 -> [w1281] mode=indexing
        tunnel: [w1283] -> w1209 mode=indexing
        tunnel: [w1284] -> w1243 mode=indexing
        tunnel: w1242 -> [w1285] mode=indexing
        tunnel: w1215 -> [w1282]
        tunnel: w1213 -> [w1277] mode=indexing
        tunnel: w1212 -> [w1276]
        tunnel: [w1273] -> w1210 mode=indexing
        w1278 = ""
        w1275 = 2 ("인덱스")
        n470 = Index Array(array=w1281, index #1=w1275) -> (element #1=w1280:string, element #2=w1279:string)  [unwired: 1 in]
        n471 = Replace Array Subset(array=w1281, new element=w1277, index=w1275) -> (w1283:string[])
        n472 = Replace Array Subset(array=w1285, new element=w1276, index=w1275) -> (w1284:string[])
        n473 = Build Array(w1282, w1282, "반시계" ("새 원소/부분배열"), w1278, w1278, w1280, w1279) -> (w1273:string[])
      }
      n474 = call "Get Spec.vi"("NumRows"=w1255, "Spec in"=w1254, "Spec Ref."=w1268, "error in"=w1229, "Condition in"=w1209, "Resolution in"=w1243, "Func_ext"=w1215) -> ("error out"=w1263:errorcluster, "Data Out"=w1211:string[][], "Func_ext Out"=w1267:string)  [unwired: 2 out]
      n475 = call "Match_CMC.vi"("CMC IN"=w1226, "error in"=w1263, "Condition IN"=w1211, "Func_ext"=w1267) -> ("error out"=w1227:errorcluster, "CMC Out"=w1208:string[][], "Func_ext out"=w1228:string)  [unwired: 4 in, 1 out]
      n476 = call "Match_CMC.vi"("CMC IN"=w1226, "error in"=w1227, "Condition IN"=w1210, "Func_ext"=w1228) -> ("error out"=w1223:errorcluster, "CMC Out"=w1220:string[][], "Func_ext out"=w1225:string)  [unwired: 4 in, 1 out]
      n477 = Index Array(array=w1220, index (col)=0 ("비활성화된 인덱스 (열)")) -> (element=w1217:string[])  [unwired: 1 in]
      n478 = Replace Array Subset(array=w1208, new element=w1217, index (col)=1 ("비활성화된 인덱스 (열)")) -> (w1207:string[][])  [unwired: 1 in]
      n479 = call "Variables Data IO.vi"("Select"=Cmd_Var_Data_IO."CMC", "error in"=w1223, "Data In"=w1207, "Func_ext"=w1225) -> ("error out"=w1222:errorcluster, "Func_ext Out"=w1224:string)  [unwired: 5 in, 1 out]
      n480 = call "Variables Data IO.vi"("Select"=Cmd_Var_Data_IO."Condition", "error in"=w1222, "Data In"=w1209, "Func_ext"=w1224) -> ("error out"=w1262:errorcluster, "Func_ext Out"=w1246:string)  [unwired: 5 in, 1 out]
      n481 = call-poly "Table Initialize.vi"("행의 개수"=w1255, "Table Ref"=w1259, "Value"=w1209, "에러 입력"=w1262) -> ("에러 출력"=w1245:errorcluster)  [unwired: 5 in, 2 out]
      n482 = Index Array(array=w1243, index (row) #1=w1235, index (col) #1=w1235, index (row) #2=w1235, index (col) #2=1 ("비활성화된 인덱스 (열)")) -> (element #1=w1234:string, element #2=w1239:string)
      n483 = Index Array(array=w1209, index (row) #1=w1261, index (col) #1=0 ("비활성화된 인덱스 (열)"), index (row) #2=w1261, index (col) #2=w1261) -> (element #1=w1250:string, element #2=w1249:string)
      n484 = Build Array(w1239) -> (w1238:string[])
      n485 = Build Array(w1250, w1249, w1234) -> (w1248:string[])
      n486 = call-poly "String Contents.vi"("문자 배열"=w1248, "참조 배열"=w1247, "에러 입력"=w1245) -> ("에러 출력"=w1241:errorcluster)  [unwired: 7 in, 1 out]
      n487 = call-poly "String Contents.vi"("문자 배열"=w1238, "참조 배열"=w1237, "에러 입력"=w1241) -> ("에러 출력"=w1240:errorcluster)  [unwired: 7 in, 1 out]
      n488 = call "Certi Recall.vi"("큐 입력"=w1258, "NumRows"=w1255, "입력 클러스터"=w1256, "에러 입력"=w1240, "Func_ext in"=w1246) -> ("에러 출력"=w1257:errorcluster)  [unwired: 5 in, 1 out]
    }
    frame Default {
    }
  }
  "data 1" <- w13
  "error out" <- w8
  n489 = Unbundle By Name(w8) -> ("status"=w2:bool)
  n490 = Not(x=w2) -> (.not. x?=→"Load?":bool)
